vi "MC_7_12b_JW.vi"() -> ()   [LabVIEW 2011]
uses:
  <vilib>/Utility/file.llb/Read From Spreadsheet File (string).vi
  <vilib>/regexp/Match Regular Expression.xnode
  <vilib>/Utility/file.llb/Write To Spreadsheet File (string).vi
  <vilib>/Utility/file.llb/Write To Spreadsheet File (DBL).vi
  <vilib>/Utility/inputDevices.llb/keyboardAcquire.vi
panel:
  out "Current \nRecord":string[](array[string])
  out "Transformer \nHeaders":string[](array[string])
  out "Current Device ID":string
  out "Column":string
  out "Row":string
  out "Concentration Recorded":string
  out "Solvent Recorded":string
  out "Method Recorded":string
  in  "?":T1(tab)
  out "Material Recorded":string
  in  "Treatment Concentration (mM):":dbl=30.0
  in  "Surface Treatment:":string
  in  "# Drops*:":dbl=inf
  in  "Solution Temp (C):":dbl=55.0
  in  "Relative Humidity (%):":dbl=nan
  in  "Room Temp (F):":dbl=nan
  in  "Time (s):":dbl=80.0
  out "Accel (RPM/s):":dbl
  in  "RPM:":dbl=1000.0
  in  "Wait Time (s):":dbl=10.0
  in  "Sample #:":dbl=1.0
  in  "Fabricator:":string="Jeremy"
  in  "Data File":path
  out "Data Folder":path
  in  "Image Folder":path
  out "Image File":path=path "D:/UserData/Desktop/Jeremy/WFU/Research/Programs/VI mods/Image Not Found.png"
  in  "Ramp (s):":dbl=3.0
  out "Cal: Trap Density-STS":dbl format="%#_4e"
  out "New: Trap Density-STS":dbl format="%#_4e"
  out "Rec: Trap Density-STS":dbl caption="Trap Density-STS" format="%#_4e"
  out "Cal: Trap Density-VT":dbl format="%#_4e"
  out "New: Trap Density-VT":dbl format="%#_4e"
  out "Rec: Trap Density-VT":dbl caption="Trap Density-VT" format="%#_4e"
  out "Calc: Onset V":dbl
  out "New: Onset":dbl
  out "Rec: Onset V":dbl caption="Onset V"
  out "Cal: Mobility-Lin":dbl format="%#_4e"
  out "New: Mobility-Lin":dbl format="%#_4e"
  out "Rec: Mobility-Lin":dbl caption="Mobility-Lin" format="%#_4e"
  out "Cal: Mobility-Sat":dbl format="%#_4e"
  out "Rec: Length":dbl caption="Length"
  out "Width":dbl
  out "Rec: Dielectric (d)":dbl caption="Dielectric (d)"
  out "XY Graph":cluster{dbl[], dbl[]}[](graph)
  in  "NumPts":dbl=5.0
  in  "Cancel Button":bool
  in  "Next Button":bool
  in  "Previous Button":bool
  in  "Up Button":bool
  in  "Down Button":bool
  out "Data Name":string
  in  "Save Changes?":bool
  in  "New Dielectric":dbl
  in  "New Length":dbl
  in  "New Width":dbl
  out "New: Mobility-Sat":dbl format="%#_4e"
  in  "Slide":dbl(slide) step=1.0 scale=-14.3..84.0 scale format="%#_1p"
  in  "Blank Button":bool
  in  "Zoom":i16(slide)=-3 scale=-5.0..5.0
  out "Image Out 2":T2(plugin-control)
  out "Image Out":T2(plugin-control)
  in  "Magnification":u16(ring) items=["5x", "10x", "20x", "50x", "80x"]
  out "Total Width":dbl
  out "Distances":dbl[](array[numeric])
  in  "Undo Button":bool
  in  "Remove Button":bool
  out "Rec: Mobility-Sat":dbl caption="Mobility-Sat" format="%#_4e"
  out "Index":string
  out "Image Name":string
  in  "Export":bool
  out "Calc: VT":dbl
  out "New: VT":dbl
  in  "Manual":bool
  out "XY Graph 2":cluster{dbl[], dbl[]}[](graph)
  in  "Next Button 2":bool
  in  "Previous Button 2":bool
  in  "Slide 2":dbl(slide) step=1.0 scale=-1.0..82.0 scale format="%#_1p"
  out "Calc: STS":dbl
  out "New: STS":dbl
  in  "NumPts 2":dbl=5.0 caption="NumPts"
  out "Rec: VT":dbl caption="Threshold V"
  out "Rec: STS":dbl caption="STS"
  out "Rec: On/Off":dbl caption="On/Off" format="%#_3e"
  in  "Save Changes? 2":bool
  in  "Save Changes? 3":bool
  out "Date Recorded":string="Date Recorded"
  out "String":string
  in  "No Image":path=path "D:/UserData/Desktop/Jeremy/WFU/Research/Programs/VI mods/Image Not Found.png"
  in  "Project":path=path "D:/UserData/Desktop/Jeremy/WFU/Research/Programs/Mega Awesome/DeviceData.opj"
  out "Index 2":dbl
  out "Array 8":dbl[](array[numeric])
  out "Array 7":dbl[](array[numeric])
  out "ROI Descriptor out":T3 {"Contours"."Type" items=["No Selection", "Point", "Line", "Rectangle", "Oval", "Polygon", "Freehand Region", "Annulus", "Unused2", "Unused3", "Broken Line", "Freehand Line", "Rotated Rectangle"]}
  out "ROI Descriptor":T3 {"Contours"."Type" items=["No Selection", "Point", "Line", "Rectangle", "Oval", "Polygon", "Freehand Region", "Annulus", "Unused2", "Unused3", "Broken Line", "Freehand Line", "Rotated Rectangle"]}
  out "Numeric 3":dbl
  out "Array 6":dbl[][](array[numeric])
  out "Cluster":T4
  out "Array 5":dbl[](array[numeric])
  out "Array 4":dbl[](array[numeric])
  out "Array 3":dbl[](array[numeric])
  out "Numeric 2":dbl
  out "Numeric":dbl
  out "Array 2":dbl[](array[numeric])
  out "Array":dbl[](array[numeric])
  out "Index":dbl
  out "Table Control 2":string[][](table)
  out "Table Control":string[][](table)
  in  "Row Start":dbl=20.0
  # "Data Locations"
  # "Data Location"
  # "Image Location"
  # "Sample Properties"
  # "*     Inf = Full coverage\n   NaN = Unknown or Not Applicable"
  # "Recorded"
  # "Calculated"
  # "Re-Calculated"
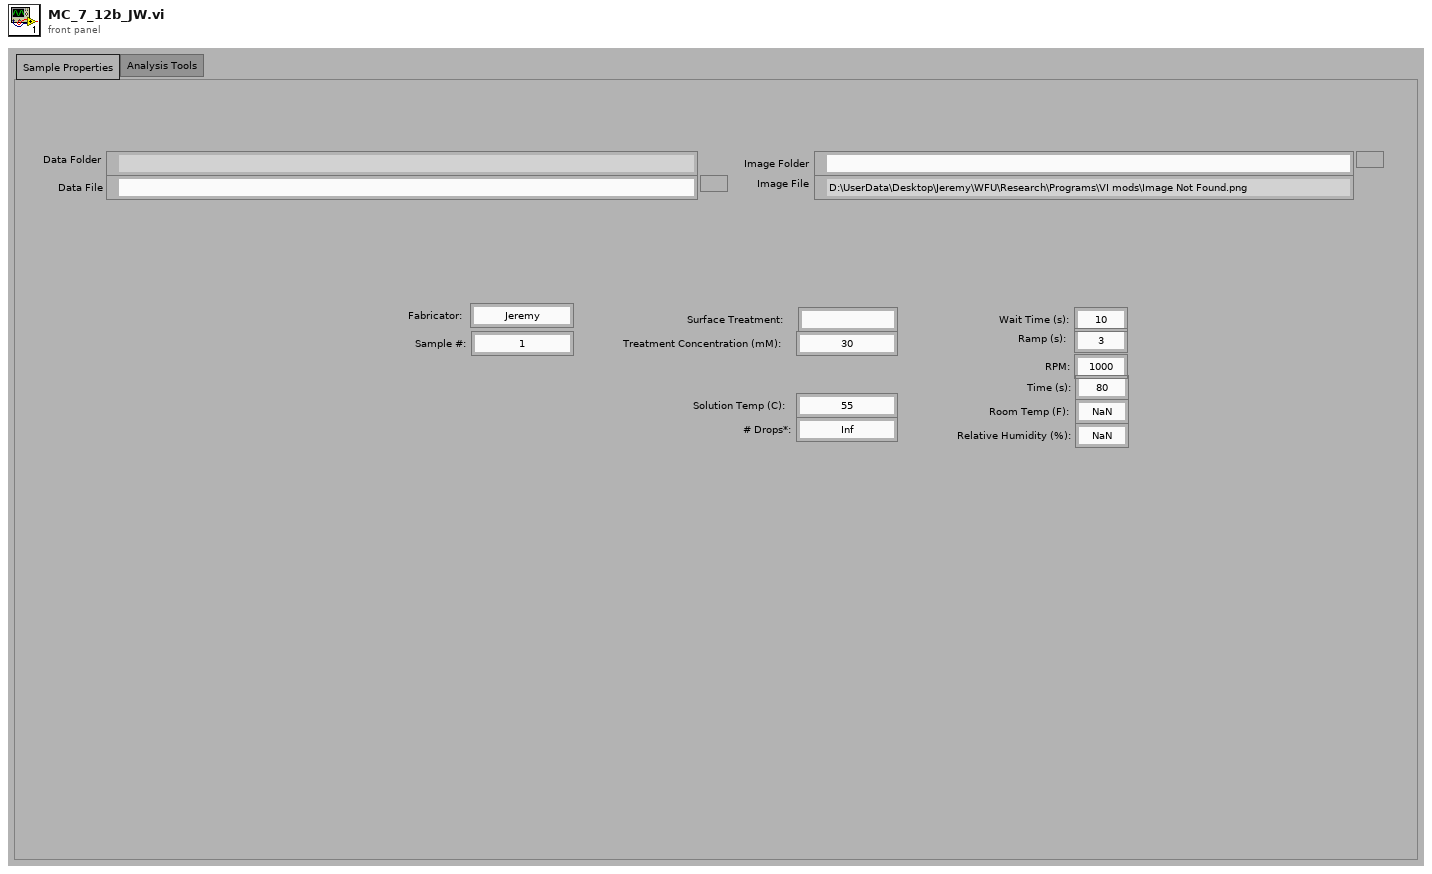
[diagram p1: front panel]
types:
  T1 = enum32{"Sample Properties", "Analysis Tools", "Current Database"}
  T2 = typedef "IMAQ Image.ctl" = refnum<image>
  T3 = typedef "ROI Descriptor" = cluster{"Global Rectangle":i32[], "Contours":cluster{"ID":enum32{"External", "Internal"}, "Type":u32, "Coordinates":i32[]}[]}
  T4 = cluster{"Numeric":dbl, "Numeric 2":dbl, "Numeric 3":dbl, "Numeric 4":dbl}
  T5 = cluster{"[0]":cluster{dbl[], dbl[]}, "[1]":cluster{dbl[], dbl[]}, "[2]":cluster{dbl[], dbl[]}, "[3]":cluster{dbl[], dbl[]}, "[4]":cluster{dbl[], dbl[]}, "[5]":cluster{dbl[], dbl[]}, "[6]":cluster{dbl[], dbl[]}, "[7]":cluster{dbl[], dbl[]}, "[8]":cluster{dbl[], dbl[]}}
  T6 = cluster{"Global Rectangle":i32[], "Contours":cluster{"Contour Type":u32, "ROI Type":u32, "Points":i32[]}[]}
  T7 = typedef "LVBoundsTypeDef.ctl" = cluster{"Width":u32, "Height":u32}
  T8 = enum16{"0", "1", "2", "3", "4", "5", "6", "7", "8", "9", "A", "B", "C", "D", "E", "F", "G", "H", "I", "J", "K", "L", "M", "N", "O", "P", "Q", "R", "S", "T", "U", "V", "W", "X", "Y", "Z", "F1", "F2", "F3", "F4", "F5", "F6", "F7", "F8", "F9", "F10", "F11", "F12", "F13", "F14", "F15", "ADD", "BACK", "BACKSLASH", "CAPITAL", "COMMA", "DECIMAL", "DELETE", "DIVIDE", "DOWN", "END", "EQUALS", "ESCAPE", "GRAVE (`)", "HOME", "INSERT", "LBRACKET", "LCONTROL", "LEFT", "L ALT", "LSHIFT", "LWIN", "MINUS", "MULTIPLY", "NEXT", "NUMLOCK", "NUMPAD_0", "NUMPAD_1", "NUMPAD_2", "NUMPAD_3", "NUMPAD_4", "NUMPAD_5", "NUMPAD_6", "NUMPAD_7", "NUMPAD_8", "NUMPAD_9", "PAUSE", "PERIOD", "PRIOR (PG UP)", "RBRACKET", "RCONTROL", "RETURN", "RIGHT", "R ALT", "RSHIFT", "RWIN", "SCROLL", "SEMICOLON", "SLASH", "SPACE", "SUBTRACT", "TAB", "UP", "ENTER (num pad)", "' (quote)"}[]
  T9 = cluster{"Contour Type":u32, "ROI Type":u32, "Points":i32[]}[]
  T10 = cluster{i32[], cluster{"Contour Type":u32, "ROI Type":u32, "Points":i32[]}[]}
  T11 = enum16{"0", "1", "2", "3", "4", "5", "6", "7", "8", "9", "A", "B", "C", "D", "E", "F", "G", "H", "I", "J", "K", "L", "M", "N", "O", "P", "Q", "R", "S", "T", "U", "V", "W", "X", "Y", "Z", "F1", "F2", "F3", "F4", "F5", "F6", "F7", "F8", "F9", "F10", "F11", "F12", "F13", "F14", "F15", "ADD", "BACK", "BACKSLASH", "CAPITAL", "COMMA", "DECIMAL", "DELETE", "DIVIDE", "DOWN", "END", "EQUALS", "ESCAPE", "GRAVE (`)", "HOME", "INSERT", "LBRACKET", "LCONTROL", "LEFT", "L ALT", "LSHIFT", "LWIN", "MINUS", "MULTIPLY", "NEXT", "NUMLOCK", "NUMPAD_0", "NUMPAD_1", "NUMPAD_2", "NUMPAD_3", "NUMPAD_4", "NUMPAD_5", "NUMPAD_6", "NUMPAD_7", "NUMPAD_8", "NUMPAD_9", "PAUSE", "PERIOD", "PRIOR (PG UP)", "RBRACKET", "RCONTROL", "RETURN", "RIGHT", "R ALT", "RSHIFT", "RWIN", "SCROLL", "SEMICOLON", "SLASH", "SPACE", "SUBTRACT", "TAB", "UP", "ENTER (num pad)", "' (quote)"}
  T12 = cluster{string, sgl, bool, bool, bool, bool, bool, bool, i32}
  T13 = cluster{i32, cluster{string, sgl, bool, bool, bool, bool, bool, bool, i32}, i32, i32}
  T14 = cluster{"Contour Type":u32, "ROI Type":u32, "Points":i32[]}
  T15 = cluster{"Points[0]":i32, "Points[1]":i32, "Points[2]":i32, "Points[3]":i32, "Points[4]":i32, "Points[5]":i32, "Points[6]":i32, "Points[7]":i32, "Points[8]":i32}
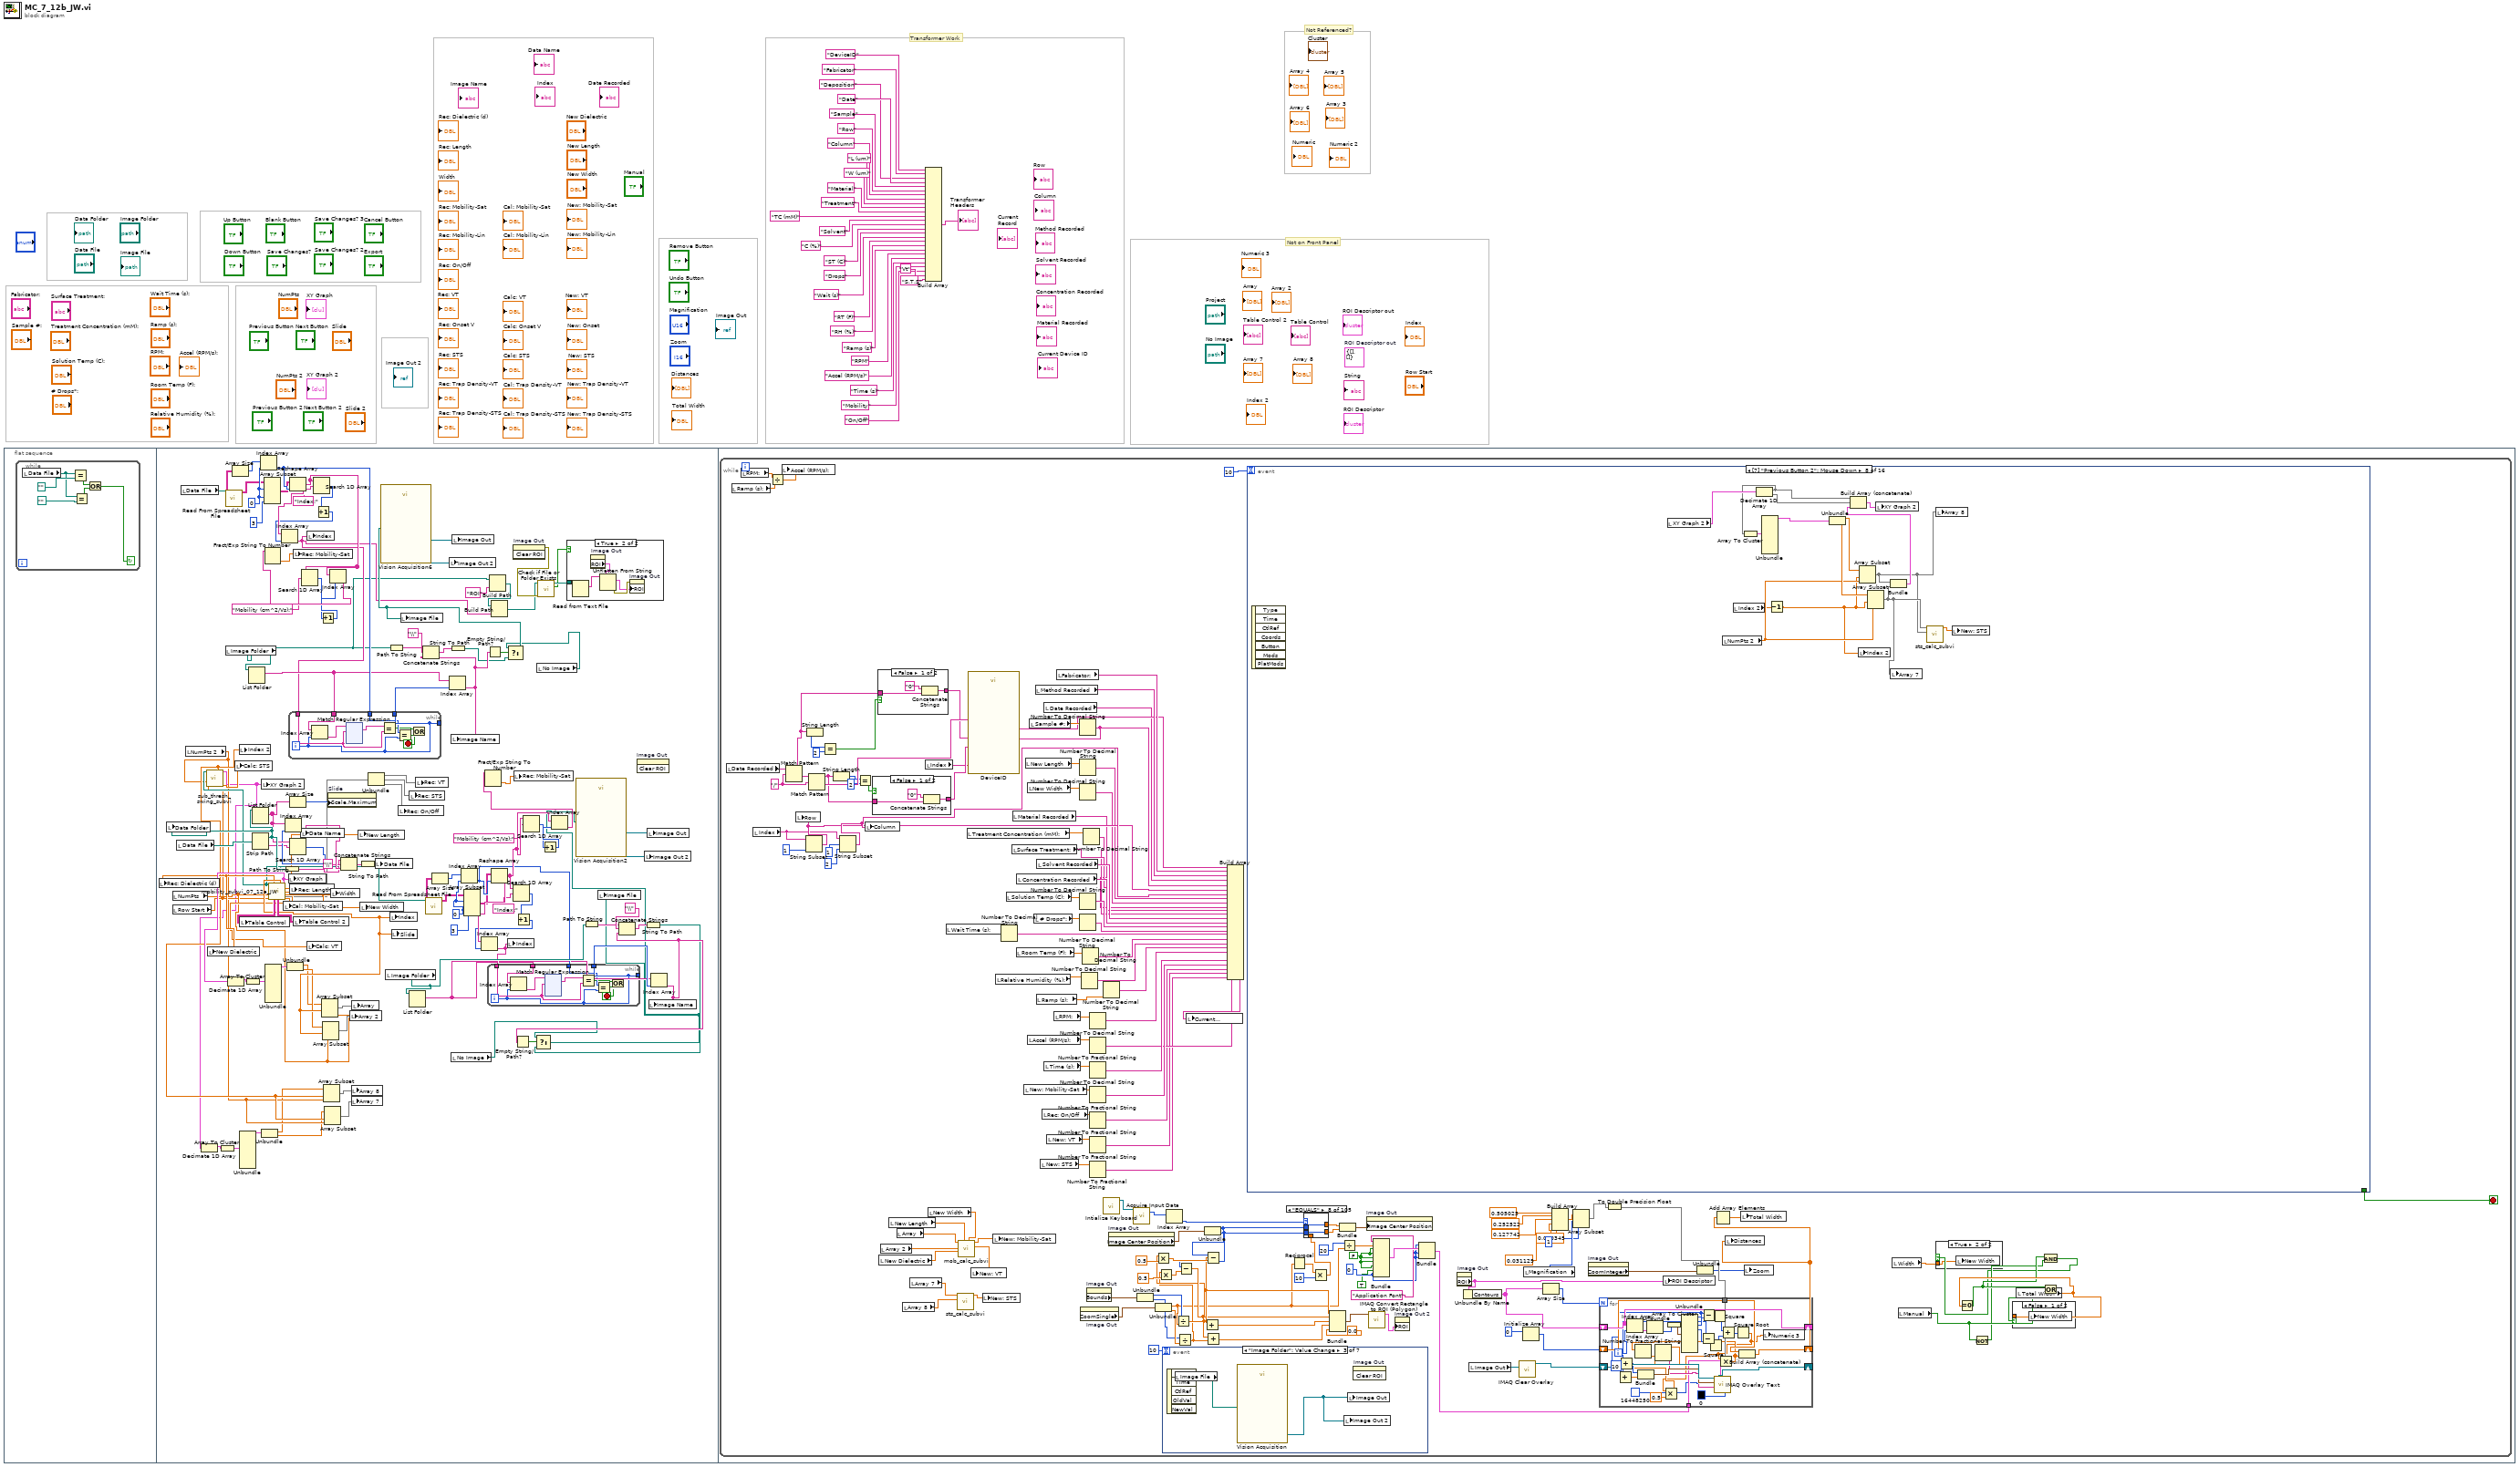
[diagram p0: block diagram]
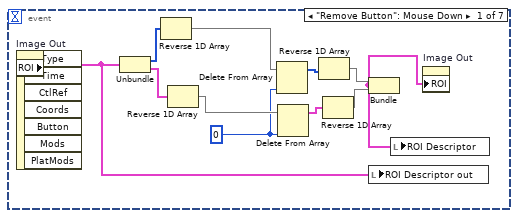
[diagram p7: hidden frame]
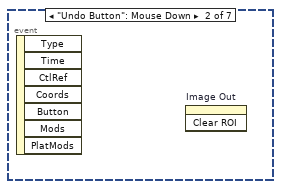
[diagram p8: hidden frame]
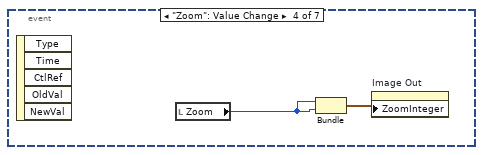
[diagram p9: hidden frame]
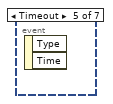
[diagram p10: hidden frame]
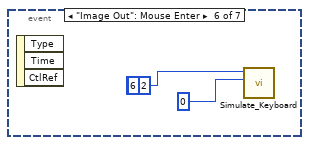
[diagram p11: hidden frame]
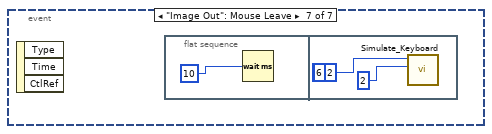
[diagram p12: hidden frame]
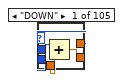
[diagram p13: hidden frame]
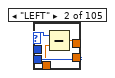
[diagram p14: hidden frame]
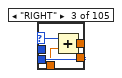
[diagram p15: hidden frame]
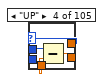
[diagram p16: hidden frame]
diagram:
  (unwired) T3 {"Global Rectangle"=[], "Contours"=[]}  # ROI Descriptor out
  # "Not Referenced?"
  # "Transformer Work"
  # "Not on Front Panel"
  n1 = flat-sequence {
    frame #0 {
      n2 = while {
        stop <- w29 continue-if-true
        n3 = local read "Data File"() -> (w31:path)
        n4 = Equal?(x=w31, y=path "") -> (x = y?=w33:bool)
        n5 = Equal?(x=w31, y=path "") -> (x = y?=w32:bool)
        n6 = Or(x=w33, y=w32) -> (x .or. y?=w29:bool)
      }
    }
    frame #1 {
      w95 = 0
      w125 = 0
      n7 = local read "NumPts"() -> (w70:dbl)
      n8 = local read "Row Start"() -> (w69:dbl)
      n9 = local read "Data File"() -> (w99:path)
      n10 = local read "Data File"() -> (w120:path)
      n11 = local read "NumPts 2"() -> (w64:dbl)
      n12 = call-poly <vilib>:"Read From Spreadsheet File.vi"("file path (dialog if empty)"=w120) -> ("all rows"=w123:string[][])  [unwired: 6 in, 4 out]
      n13 = local read "Image Folder"() -> (w35:path)
      n14 = Array Size(array=w123) -> (size(s)=w124:i32[])
      n15 = List Folder(path=w35) -> (filenames=w129:string[])  [unwired: 3 in, 3 out]
      n16 = Strip Path(path=w99) -> (stripped path=w100:path, name=w81:string)
      n17 = local write "Data Folder"(w100) -> ()
      n18 = List Folder(path=w100) -> (filenames=w89:string[])  [unwired: 3 in, 3 out]
      n19 = Index Array(array=w124, index=w125) -> (element=w131:i32)
      n20 = Array Subset(array=w123, index (row)=w125, index (col)=w125, length (col)=3) -> (w122:string[][])  [unwired: 1 in]
      n21 = Path To String(path=w100) -> (string=w80:string)
      n22 = Reshape Array(w122, w131) -> (w141:string[])
      n23 = Array Size(array=w89) -> (size(s)=w90:i32)
      n24 = Search 1D Array(1D array=w89, element=w81) -> (index of element=w88:i32)  [unwired: 1 in]
      n25 = Index Array(array=w89, index=w88) -> (element=w87:string)
      n26 = local write "Data Name"(w87) -> ()
      n27 = Search 1D Array(1D array=w141, element="Mobility (cm^2/Vs):") -> (index of element=w136:i32)  [unwired: 1 in]
      n28 = Search 1D Array(1D array=w141, element="Index:") -> (index of element=w128:i32)  [unwired: 1 in]
      n29 = Increment(x=w128) -> (x+1=w127:i32)
      n30 = Index Array(array=w141, index=w127) -> (element=w36:string)
      n31 = while {
        tunnel: w129 -> [w274]
        tunnel: w36 -> [w272]
        tunnel: [w271] -> _
        tunnel: [w271] -> w130
        tunnel: w131 -> [w270]
        i -> [w271]
        stop <- w267 stop-if-true
        n32 = Index Array(array=w274, index=w271) -> (element=w275:string)
        n33 = xnode "Match Regular Expression"("input string"=w275, "regular expression"=w272) -> ("whole match"=w273:string)  [unwired: 4 in, 4 out]
        n34 = Equal?(x=w273, y=w272) -> (x = y?=w269:bool)
        n35 = Equal?(x=w270, y=w271) -> (x = y?=w268:bool)
        n36 = Or(x=w269, y=w268) -> (x .or. y?=w267:bool)
      }
      n37 = local write "Index"(w36) -> ()
      n38 = Increment(x=w136) -> (x+1=w137:i32)
      n39 = property on="Slide" class="Slide (strict)"("Scale.Maximum"=w90) -> ()  [unwired: 2 in, 2 out]
      n40 = Index Array(array=w141, index=w137) -> (element=w139:string)
      n41 = Fract/Exp String To Number(string=w139) -> (number=w140:dbl)  [unwired: 3 in, 1 out]
      n42 = local write "Rec: Mobility-Sat"(w140) -> ()
      n43 = Concatenate Strings(w80, "\\", w87) -> (w82:string)
      n44 = String To Path(string=w82) -> (path=w71:path)
      n45 = call "sub_thresh_swing_subvi.vi"("Path"=w71, "NumPts"=w64, "Row Start"=w69) -> ("Index"=w65:dbl, "XY Graph"=w60:cluster{dbl[], dbl[]}[], "Sub Threshold Swing"=w72:dbl)  [unwired: 8 in, 2 out]
      n46 = Decimate 1D Array(w60) -> (w61:cluster{dbl[], dbl[]}[])  [unwired: 1 out]
      n47 = Array To Cluster(array=w61) -> (cluster=w63:T5)
      n48 = local write "Calc: STS"(w72) -> ()
      n49 = local write "Index 2"(w65) -> ()
      n50 = Unbundle(w63) -> ("[0]"=w62:cluster{dbl[], dbl[]})  [unwired: 8 out]
      n51 = local write "XY Graph 2"(w60) -> ()
      n52 = Unbundle(w62) -> (w58:dbl[], w57:dbl[])
      n53 = call "mobility_subvi_07_12a_JW.vi"("Path"=w71, "NumPts"=w70, 11:w69) -> ("Dielectric (d)"=w76:dbl, "Index"=w77:dbl, "XY Graph"=w119:cluster{dbl[], dbl[]}[], "Length"=w75:dbl, "Vt"=w73:dbl, "Width"=w74:dbl, "Table Control"=w84:string[][], "Table Control 2"=w85:string[][], 14:w54, "Mobility"=w86:dbl)  [unwired: 2 in, 1 out]
      n54 = local write "Rec: Dielectric (d)"(w76) -> ()
      n55 = local write "New Dielectric"(w76) -> ()
      n56 = Decimate 1D Array(w119) -> (w118:cluster{dbl[], dbl[]}[])  [unwired: 1 out]
      n57 = local write "Table Control"(w84) -> ()
      n58 = Array To Cluster(array=w118) -> (cluster=w116:T5)
      n59 = Unbundle(w116) -> ("[0]"=w117:cluster{dbl[], dbl[]})  [unwired: 8 out]
      n60 = local write "Cal: Mobility-Sat"(w86) -> ()
      n61 = Unbundle(w117) -> (w59:dbl[], w66:dbl[])
      n62 = local write "XY Graph"(w119) -> ()
      n63 = local write "Rec: Length"(w75) -> ()
      n64 = local write "Table Control 2"(w85) -> ()
      n65 = local write "Calc: VT"(w73) -> ()
      n66 = Array Subset(array=w59, index=w77, length=w70) -> (w78:dbl[])
      n67 = Array Subset(array=w66, index=w77, length=w70) -> (w79:dbl[])
      n68 = Array Subset(array=w58, index=w65, length=w64) -> (w68:dbl[])
      n69 = Array Subset(array=w57, index=w65, length=w64) -> (w67:dbl[])
      n70 = local write "Width"(w74) -> ()
      n71 = local write "Array 2"(w79) -> ()
      n72 = local write "Array 8"(w68) -> ()
      n73 = local write "Array 7"(w67) -> ()
      n74 = local write "Array"(w78) -> ()
      n75 = local write "New Length"(w75) -> ()
      n76 = local write "New Width"(w74) -> ()
      n77 = Unbundle(w54) -> ("Vt"=w56, "STS"=w55, "On/Off"=w53)
      n78 = local write "Data File"(w71) -> ()
      n79 = local read "Image Folder"() -> (w106:path)
      n80 = Path To String(path=w35) -> (string=w133:string)
      n81 = local write "Index"(w77) -> ()
      n82 = local write "Slide"(w77) -> ()
      n83 = local write "Rec: On/Off"(w53) -> ()
      n84 = List Folder(path=w106) -> (filenames=w102:string[])  [unwired: 3 in, 3 out]
      n85 = local write "Rec: STS"(w55) -> ()
      n86 = local write "Rec: VT"(w56) -> ()
      n87 = call-poly <vilib>:"Read From Spreadsheet File.vi"("file path (dialog if empty)"=w71) -> ("all rows"=w93:string[][])  [unwired: 6 in, 4 out]
      n88 = Array Size(array=w93) -> (size(s)=w94:i32[])
      n89 = Index Array(array=w129, index=w130) -> (element=w52:string)
      n90 = Concatenate Strings(w133, "\\", w52) -> (w134:string)
      n91 = String To Path(string=w134) -> (path=w50:path)
      n92 = local write "Image Name"(w52) -> ()
      n93 = local read "No Image"() -> (w44:path)
      n94 = Index Array(array=w94, index=w95) -> (element=w105:i32)
      n95 = Array Subset(array=w93, index (row)=w95, index (col)=w95, length (col)=3) -> (w92:string[][])  [unwired: 1 in]
      n96 = Empty String/Path?(string/path=w52) -> (empty?=w51:bool)
      n97 = Build Path(base path=w35, name or relative path="ROI") -> (appended path=w38:path)
      n98 = Build Path(base path=w38, name or relative path=w36) -> (appended path=w37:path)
      n99 = Reshape Array(w92, w105) -> (w115:string[])
      n100 = invoke on="Image Out" class="ImageControl" method="Clear ROI"() -> (error out=w42:errorcluster)  [unwired: 3 in, 2 out]
      n101 = Search 1D Array(1D array=w115, element="Index:") -> (index of element=w98:i32)  [unwired: 1 in]
      n102 = Increment(x=w98) -> (x+1=w97:i32)
      n103 = Index Array(array=w115, index=w97) -> (element=w103:string)
      n104 = while {
        tunnel: w102 -> [w154]
        tunnel: w103 -> [w152]
        tunnel: [w151] -> _
        tunnel: [w151] -> w104
        tunnel: w105 -> [w150]
        i -> [w151]
        stop <- w147 stop-if-true
        n105 = Index Array(array=w154, index=w151) -> (element=w155:string)
        n106 = xnode "Match Regular Expression"("input string"=w155, "regular expression"=w152) -> ("whole match"=w153:string)  [unwired: 4 in, 4 out]
        n107 = Equal?(x=w153, y=w152) -> (x = y?=w149:bool)
        n108 = Equal?(x=w150, y=w151) -> (x = y?=w148:bool)
        n109 = Or(x=w149, y=w148) -> (x .or. y?=w147:bool)
      }
      n110 = local write "Index"(w103) -> ()
      n111 = Search 1D Array(1D array=w115, element="Mobility (cm^2/Vs):") -> (index of element=w110:i32)  [unwired: 1 in]
      n112 = local read "No Image"() -> (w43:path)
      n113 = Select(t=w43, s=w51, f=w50) -> (s? t:f=w49:path)
      n114 = call "Vision Acquisition6"("Image Path"=w49) -> ("Image Out"=w132:T2)  [unwired: 25 in, 1 out]
      n115 = local write "Image File"(w49) -> ()
      n116 = local write "Image Out 2"(w132) -> ()
      n117 = local write "Image Out"(w132) -> ()
      n118 = call <vilib>:"Check if File or Folder Exists.vi"("error in (no error)"=w42, "path"=w37) -> ("file or folder exists?"=w40:bool, "dup path"=w41:path)  [unwired: 7 in, 1 out]
      n119 = Increment(x=w110) -> (x+1=w111:i32)
      n120 = Index Array(array=w115, index=w111) -> (element=w113:string)
      n121 = Fract/Exp String To Number(string=w113) -> (number=w114:dbl)  [unwired: 3 in, 1 out]
      n122 = local write "Rec: Mobility-Sat"(w114) -> ()
      n123 = case shown="True" w40 {
        tunnel: w41 -> [_ w142]
        frame False {
        }
        frame True {
          n124 = Read from Text File(file (use dialog)=w142) -> (text=w146:string)  [unwired: 3 in, 3 out]
          n125 = property on="Image Out" class="ImageControl"() -> ("ROI"=w143:T6)  [unwired: 2 in, 2 out]
          n126 = Unflatten From String(type=w143, binary string=w146) -> (value=w144:T6, error out=w145:errorcluster)  [unwired: 3 in, 1 out]
          n127 = property on="Image Out" class="ImageControl"(error in=w145, "ROI"=w144) -> ()  [unwired: 1 in, 2 out]
        }
      }
      n128 = Path To String(path=w106) -> (string=w107:string)
      n129 = invoke on="Image Out" class="ImageControl" method="Clear ROI"() -> ()  [unwired: 3 in, 3 out]
      n130 = Index Array(array=w102, index=w104) -> (element=w47:string)
      n131 = Empty String/Path?(string/path=w47) -> (empty?=w48:bool)
      n132 = Concatenate Strings(w107, "\\", w47) -> (w108:string)
      n133 = String To Path(string=w108) -> (path=w46:path)
      n134 = Select(t=w44, s=w48, f=w46) -> (s? t:f=w45:path)
      n135 = call "Vision Acquisition2"("Image Path"=w45) -> ("Image Out"=w101:T2)  [unwired: 25 in, 1 out]
      n136 = local write "Image File"(w45) -> ()
      n137 = local write "Image Out 2"(w101) -> ()
      n138 = local write "Image Out"(w101) -> ()
      n139 = local write "Image Name"(w47) -> ()
    }
    frame #2 {
      n140 = while {
        stop <- w533 stop-if-true
        w419 = "/"
        w483 = FALSE
        w481 = 0
        n141 = local read "Date Recorded"() -> (w422:string)
        n142 = local read "Ramp (s):"() -> (w388:dbl)
        n143 = local read "RPM:"() -> (w389:dbl)
        n144 = local read "Index"() -> (w391:string)
        n145 = Divide(x=w389, y=w388) -> (x/y=w387:dbl)
        n146 = local write "Accel (RPM/s):"(w387) -> ()
        n147 = Match Pattern(string=w422, regular expression=w419) -> (before substring=w413:string, after substring=w420:string)  [unwired: 1 in, 2 out]
        n148 = String Subset(string=w391, length (rest)=1) -> (substring=w447:string)  [unwired: 1 in]
        n149 = local write "Row"(w447) -> ()
        n150 = String Length(string=w413) -> (length=w416:i32)
        n151 = Match Pattern(string=w420, regular expression=w419) -> (before substring=w407:string, after substring=w418:string)  [unwired: 1 in, 2 out]
        n152 = Equal?(x=w416, y=2) -> (x = y?=w414:bool)
        n153 = String Length(string=w407) -> (length=w409:i32)
        n154 = String Subset(string=w391, offset (0)=1, length (rest)=2) -> (substring=w448:string)
        n155 = Equal?(x=w409, y=2) -> (x = y?=w411:bool)
        n156 = local write "Column"(w448) -> ()
        n157 = case shown="False" w411 {
          tunnel: w407 -> [w535 w537]
          tunnel: [w534 w537] -> w408
          frame False {
            n158 = Concatenate Strings("0", w535) -> (w534:string)
          }
          frame True {
          }
        }
        n159 = case shown="False" w414 {
          tunnel: w413 -> [w539 w541]
          tunnel: [w538 w541] -> w412
          frame False {
            n160 = Concatenate Strings("0", w539) -> (w538:string)
          }
          frame True {
          }
        }
        n161 = local read "New Dielectric"() -> (w471:dbl)
        n162 = local read "Array 2"() -> (w467:dbl[])
        n163 = local read "New Length"() -> (w469:dbl)
        n164 = local read "Array"() -> (w468:dbl[])
        n165 = local read "Array 8"() -> (w463:dbl[])
        n166 = local read "Array 7"() -> (w464:dbl[])
        n167 = local read "Index"() -> (w406:string)
        n168 = local read "New Width"() -> (w472:dbl)
        n169 = local read "Wait Time (s):"() -> (w452:dbl)
        n170 = call "sts_calc_subvi.vi"("Array 2"=w463, "Array"=w464) -> ("STS"=w465:dbl)  [unwired: 9 in]
        n171 = call "mob_calc_subvi.vi"("Width"=w472, "Length"=w469, "Dielectric (d)"=w471, "Array 2"=w467, "Array"=w468) -> ("Vt"=w466:dbl, "Mobility"=w470:dbl)  [unwired: 4 in, 1 out]
        n172 = local read "Treatment Concentration (mM):"() -> (w399:dbl)
        n173 = local write "New: VT"(w466) -> ()
        n174 = local write "New: STS"(w465) -> ()
        n175 = local write "New: Mobility-Sat"(w470) -> ()
        n176 = local read "Relative Humidity (%):"() -> (w396:dbl)
        n177 = Number To Decimal String(number=w452) -> (decimal integer string=w453:string)  [unwired: 1 in]
        n178 = local read "Solution Temp (C):"() -> (w441:dbl)
        n179 = local read "Surface Treatment:"() -> (w398:string)
        n180 = local read "Material Recorded"() -> (w394:string)
        n181 = local read "Room Temp (F):"() -> (w445:dbl)
        n182 = local read "Concentration Recorded"() -> (w401:string)
        n183 = local read "New: Mobility-Sat"() -> (w434:dbl)
        n184 = local read "New Length"() -> (w405:dbl)
        n185 = local read "New Width"() -> (w404:dbl)
        n186 = local read "Accel (RPM/s):"() -> (w432:dbl)
        n187 = local read "Sample #:"() -> (w424:dbl)
        n188 = local read "# Drops*:"() -> (w442:dbl)
        n189 = local read "Method Recorded"() -> (w425:string)
        n190 = local read "Ramp (s):"() -> (w450:dbl)
        n191 = local read "Solvent Recorded"() -> (w400:string)
        n192 = local read "New: STS"() -> (w426:dbl)
        n193 = local read "Rec: On/Off"() -> (w430:dbl)
        n194 = local read "Date Recorded"() -> (w421:string)
        n195 = local read "Time (s):"() -> (w437:dbl)
        n196 = local read "New: VT"() -> (w428:dbl)
        n197 = local read "RPM:"() -> (w438:dbl)
        n198 = local read "Fabricator:"() -> (w446:string)
        n199 = Number To Decimal String(number=w442) -> (decimal integer string=w443:string)  [unwired: 1 in]
        n200 = Number To Decimal String(number=w424) -> (decimal integer string=w417:string)  [unwired: 1 in]
        n201 = call "DeviceID"("Sample"=w417, "Year"=w418, "Month"=w412, "Day"=w408, "Index"=w406) -> ("Result"=w423:string)  [unwired: 9 in, 1 out]
        n202 = Number To Decimal String(number=w405) -> (decimal integer string=w403:string)  [unwired: 1 in]
        n203 = Number To Decimal String(number=w404) -> (decimal integer string=w402:string)  [unwired: 1 in]
        n204 = Number To Decimal String(number=w441) -> (decimal integer string=w440:string)  [unwired: 1 in]
        n205 = property on="Image Out" class="ImageControl"() -> ("ZoomSingle"=w501:cluster{"X":sgl, "Y":sgl})  [unwired: 2 in, 2 out]
        n206 = Number To Decimal String(number=w396) -> (decimal integer string=w395:string)  [unwired: 1 in]
        n207 = Number To Decimal String(number=w445) -> (decimal integer string=w444:string)  [unwired: 1 in]
        n208 = Number To Decimal String(number=w399) -> (decimal integer string=w397:string)  [unwired: 1 in]
        n209 = property on="Image Out" class="ImageControl"() -> ("Bounds"=w502:T7)  [unwired: 2 in, 2 out]
        n210 = Number To Decimal String(number=w438) -> (decimal integer string=w439:string)  [unwired: 1 in]
        n211 = Number To Fractional String(number=w432) -> (F-format string=w433:string)  [unwired: 3 in]
        n212 = Number To Decimal String(number=w437) -> (decimal integer string=w436:string)  [unwired: 1 in]
        n213 = Number To Fractional String(number=w434) -> (F-format string=w435:string)  [unwired: 3 in]
        n214 = Number To Fractional String(number=w430) -> (F-format string=w431:string)  [unwired: 3 in]
        n215 = Number To Fractional String(number=w428) -> (F-format string=w429:string)  [unwired: 3 in]
        n216 = Number To Fractional String(number=w426) -> (F-format string=w427:string)  [unwired: 3 in]
        n217 = Number To Decimal String(number=w450) -> (decimal integer string=w451:string)  [unwired: 1 in]
        n218 = call <vilib>:"Intialize Keyboard.vi"() -> ("device ID"=w513:refnum<k1>)  [unwired: 10 in, 1 out]
        n219 = property on="Image Out" class="ImageControl"() -> ("Image Center Position"=w508:cluster{"X":u32, "Y":u32})  [unwired: 2 in, 2 out]
        n220 = call-poly <vilib>:"Acquire Input Data.vi"("device ID"=w513) -> ("keys pressed"=w512:T8)  [unwired: 16 in, 2 out]
        n221 = Unbundle(w502) -> ("Width"=w499:u32, "Height"=w498:u32)
        n222 = Unbundle(w501) -> ("X"=w476:sgl, "Y"=w500:sgl)
        n223 = event shown="[2] \" Image Folder\": Value Change" {
          selector: _ -> [_ _ _ _ _ _ _]
          dyn-events: _ -> [_ _ _ _ _ _ _]
          timeout: 10 -> [_ _ _ _ _ _ _]
          event "Remove Button": Mouse Down {
            w546 = 0
            n224 = property on="Image Out" class="ImageControl"() -> ("ROI"=w544:T6)  [unwired: 2 in, 2 out]
            n225 = event-data() -> ()  [unwired: 1 in, 7 out]
            n226 = Unbundle(w544) -> ("Global Rectangle"=w547:i32[], "Contours"=w549:T9)
            n227 = Reverse 1D Array(array=w547) -> (reversed array=w548:i32[])
            n228 = Reverse 1D Array(array=w549) -> (reversed array=w550:T9)
            n229 = Delete From Array(array=w548, index=w546) -> (array with subset deleted=w551:i32[])  [unwired: 1 in, 1 out]
            n230 = Delete From Array(array=w550, index=w546) -> (array with subset deleted=w552:T9)  [unwired: 1 in, 1 out]
            n231 = Reverse 1D Array(array=w551) -> (reversed array=w553:i32[])
            n232 = Reverse 1D Array(array=w552) -> (reversed array=w554:T9)
            n233 = Bundle(w553, w554) -> (w545:T10)  [unwired: 1 in]
            n234 = local write "ROI Descriptor out"(w544) -> ()
            n235 = local write "ROI Descriptor"(w545) -> ()
            n236 = property on="Image Out" class="ImageControl"("ROI"=w545) -> ()  [unwired: 2 in, 2 out]
          }
          event "Undo Button": Mouse Down {
            n237 = event-data() -> ()  [unwired: 1 in, 7 out]
            n238 = invoke on="Image Out" class="ImageControl" method="Clear ROI"() -> ()  [unwired: 3 in, 3 out]
          }
          event "Image Folder": Value Change {
            n239 = event-data() -> ()  [unwired: 1 in, 5 out]
            n240 = local read "Image File"() -> (w556:path)
            n241 = call "Vision Acquisition"("Image Path"=w556) -> ("Image Out"=w555:T2)  [unwired: 25 in, 1 out]
            n242 = local write "Image Out 2"(w555) -> ()
            n243 = local write "Image Out"(w555) -> ()
            n244 = invoke on="Image Out" class="ImageControl" method="Clear ROI"() -> ()  [unwired: 3 in, 3 out]
          }
          event "Zoom": Value Change {
            n245 = event-data() -> ()  [unwired: 1 in, 5 out]
            n246 = local read "Zoom"() -> (w557:i16)
            n247 = Bundle("Zoom"=w557, "Zoom"=w557) -> (w558:cluster{"Zoom":i16, "Zoom":i16})  [unwired: 1 in]
            n248 = property on="Image Out" class="ImageControl"("ZoomInteger"=w558) -> ()  [unwired: 2 in, 2 out]
          }
          event Timeout {
            n249 = event-data() -> ()  [unwired: 1 in, 2 out]
          }
          event "Image Out": Mouse Enter {
            (unwired) 6
            n250 = event-data() -> ()  [unwired: 1 in, 3 out]
            n251 = call "Simulate_Keyboard.vi"("Action"=0, "Virtual Key"=162) -> ()  [unwired: 7 in, 1 out]
          }
          event "Image Out": Mouse Leave {
            n252 = event-data() -> ()  [unwired: 1 in, 3 out]
            n253 = flat-sequence {
              frame #0 {
                n254 = Wait (ms)(milliseconds to wait=10) -> ()  [unwired: 1 out]
              }
              frame #1 {
                (unwired) 6
                n255 = call "Simulate_Keyboard.vi"("Action"=2, "Virtual Key"=162) -> ()  [unwired: 7 in, 1 out]
              }
            }
          }
        }
        n256 = Index Array(array=w512) -> (element=w516:T11)  [unwired: 1 in]
        n257 = Divide(x=w499, y=w476) -> (x/y=w489:sgl)
        n258 = Multiply(x=w489, y=0.5) -> (x*y=w495:dbl)
        n259 = Divide(x=w498, y=w500) -> (x/y=w488:sgl)
        n260 = Multiply(x=w488, y=0.5) -> (x*y=w494:dbl)
        n261 = Unbundle(w508) -> ("X"=w490:u32, "Y"=w491:u32)
        n262 = Subtract(x=w491, y=w494) -> (x-y=w492:dbl)
        n263 = Subtract(x=w490, y=w495) -> (x-y=w493:dbl)
        n264 = Add(x=w493, y=w489) -> (x+y=w507:dbl)
        n265 = Add(x=w492, y=w488) -> (x+y=w506:dbl)
        n266 = Build Array(w423, w446, w425, w421, w417, w447, w448, w403, w402, w394, w398, w397, w400, w401, w440, w443, w453, w444, w395, w451, w439, w433, w436, w435, w431, w429, w427) -> (w449:string[])
        n267 = local write "Current \nRecord"(w449) -> ()
        n268 = event shown="[7] \"Previous Button 2\": Mouse Down" {
          selector: _ -> [_ _ _ _ _ _ _ _ _ _ _ _ _ _ _ _]
          dyn-events: _ -> [_ _ _ _ _ _ _ _ _ _ _ _ _ _ _ _]
          timeout: 10 -> [_ _ _ _ _ _ _ _ _ _ _ _ _ _ _ _]
          tunnel: [_ _ _ _ _ _ _ _ _ _ _ _ _ TRUE _ TRUE] -> w533
          event Timeout {
            n269 = event-data() -> ()  [unwired: 1 in, 2 out]
          }
          event "Down Button": Mouse Down {
            w889 = 0
            n270 = event-data() -> ()  [unwired: 1 in, 7 out]
            n271 = local read "NumPts 2"() -> (w850:dbl)
            n272 = local read "NumPts"() -> (w857:dbl)
            n273 = local read "Row Start"() -> (w856:dbl)
            n274 = local read "Data File"() -> (w894:path)
            n275 = property on="Image Out" class="ImageControl"() -> (error out=w819:errorcluster, "Image Center Position"=w823:cluster{"X":u32, "Y":u32})  [unwired: 2 in, 1 out]
            n276 = Strip Path(path=w894) -> (stripped path=w885:path, name=w907:string)
            n277 = local write "Data Folder"(w885) -> ()
            n278 = List Folder(path=w885) -> (filenames=w900:string[], error out=w828:errorcluster)  [unwired: 3 in, 2 out]
            n279 = Array Size(array=w900) -> (size(s)=w895:i32)
            n280 = Path To String(path=w885) -> (string=w908:string)
            n281 = Search 1D Array(1D array=w900, element=w907) -> (index of element=w897:i32)  [unwired: 1 in]
            n282 = Unbundle(w823) -> ("X"=w821:u32)  [unwired: 1 out]
            n283 = Bundle("X"=w821, 0) -> (w822:cluster{"X":u32, i32})  [unwired: 1 in]
            n284 = Decrement(x=w895) -> (x-1=w898:i32)
            n285 = Equal?(x=w897, y=w898) -> (x = y?=w899:bool)
            n286 = case shown="False" w899 {
              tunnel: w897 -> [w1035 _]
              tunnel: [w1034 0] -> w896
              frame False {
                n287 = Increment(x=w1035) -> (x+1=w1034:i32)
              }
              frame True {
              }
            }
            n288 = Index Array(array=w900, index=w896) -> (element=w901:string)
            n289 = local write "Data Name"(w901) -> ()
            n290 = Concatenate Strings(w908, "\\", w901) -> (w906:string)
            n291 = property on="Image Out" class="ImageControl"(error in=w819, "Image Center Position"=w822) -> ()  [unwired: 1 in, 2 out]
            n292 = String To Path(string=w906) -> (path=w858:path)
            n293 = call "sub_thresh_swing_subvi.vi"("Path"=w858, "NumPts"=w850, "Row Start"=w856) -> ("Index"=w851:dbl, "XY Graph"=w846:cluster{dbl[], dbl[]}[], "Sub Threshold Swing"=w859:dbl)  [unwired: 8 in, 2 out]
            n294 = Decimate 1D Array(w846) -> (w849:cluster{dbl[], dbl[]}[])  [unwired: 1 out]
            n295 = Array To Cluster(array=w849) -> (cluster=w847:T5)
            n296 = Unbundle(w847) -> ("[0]"=w848:cluster{dbl[], dbl[]})  [unwired: 8 out]
            n297 = Unbundle(w848) -> (w845:dbl[], w844:dbl[])
            n298 = local write "Calc: STS"(w859) -> ()
            n299 = local write "XY Graph 2"(w846) -> ()
            n300 = local write "Index 2"(w851) -> ()
            n301 = call "mobility_subvi_07_12a_JW.vi"("Path"=w858, "NumPts"=w857, 11:w856) -> ("Dielectric (d)"=w861:dbl, "Capacitance (C)"=w818:dbl, "Index"=w866:dbl, "XY Graph"=w869:cluster{dbl[], dbl[]}[], "Length"=w860:dbl, "Vt"=w862:dbl, "Width"=w834:dbl, "Table Control"=w904:string[][], "Table Control 2"=w903:string[][], 14:w843, "Mobility"=w902:dbl)  [unwired: 2 in]
            n302 = local write "Rec: Dielectric (d)"(w861) -> ()
            n303 = local write "Calc: VT"(w862) -> ()
            n304 = local write "New Dielectric"(w861) -> ()
            n305 = Decimate 1D Array(w869) -> (w870:cluster{dbl[], dbl[]}[])  [unwired: 1 out]
            n306 = Array To Cluster(array=w870) -> (cluster=w872:T5)
            n307 = local write "Table Control"(w904) -> ()
            n308 = Unbundle(w872) -> ("[0]"=w871:cluster{dbl[], dbl[]})  [unwired: 8 out]
            n309 = Unbundle(w871) -> (w853:dbl[], w852:dbl[])
            n310 = local write "Cal: Mobility-Sat"(w902) -> ()
            n311 = local write "XY Graph"(w869) -> ()
            n312 = local write "Table Control 2"(w903) -> ()
            n313 = Array Subset(array=w853, index=w866, length=w857) -> (w868:dbl[])
            n314 = Array Subset(array=w852, index=w866, length=w857) -> (w867:dbl[])
            n315 = Unbundle(w843) -> (w842, w841, w840, w817, w816, w815, w814)
            n316 = local write "Rec: On/Off"(w840) -> ()
            n317 = local write "Rec: Length"(w860) -> ()
            n318 = local write "Width"(w834) -> ()
            n319 = local write "Array 2"(w867) -> ()
            n320 = local write "Array"(w868) -> ()
            n321 = local write "Slide"(w866) -> ()
            n322 = local write "Index"(w866) -> ()
            n323 = local write "Date Recorded"(w818) -> ()
            n324 = local write "Rec: STS"(w841) -> ()
            n325 = local write "Solvent Recorded"(w816) -> ()
            n326 = local write "Concentration Recorded"(w815) -> ()
            n327 = local write "Method Recorded"(w817) -> ()
            n328 = local write "Rec: VT"(w842) -> ()
            n329 = Array Subset(array=w845, index=w851, length=w850) -> (w855:dbl[])
            n330 = Array Subset(array=w844, index=w851, length=w850) -> (w854:dbl[])
            n331 = local write "New Width"(w834) -> ()
            n332 = local write "Material Recorded"(w814) -> ()
            n333 = local write "Data File"(w858) -> ()
            n334 = local write "New Length"(w860) -> ()
            n335 = local write "Array 8"(w855) -> ()
            n336 = local write "Array 7"(w854) -> ()
            n337 = call-poly <vilib>:"Read From Spreadsheet File.vi"("file path (dialog if empty)"=w858) -> ("all rows"=w891:string[][])  [unwired: 6 in, 4 out]
            n338 = local read "Image Folder"() -> (w825:path)
            n339 = Array Size(array=w891) -> (size(s)=w890:i32[])
            n340 = List Folder(path=w825, error in=w828) -> (filenames=w884:string[], error out=w829:errorcluster)  [unwired: 2 in, 2 out]
            n341 = Index Array(array=w890, index=w889) -> (element=w864:i32)
            n342 = Subtract(x=w864, y=20) -> (x-y=w863:i32)
            n343 = property on="Slide" class="Slide (strict)"("Scale.Maximum"=w863) -> ()  [unwired: 2 in, 2 out]
            n344 = Array Subset(array=w891, index (row)=w889, index (col)=w889, length (col)=3) -> (w892:string[][])  [unwired: 1 in]
            n345 = Reshape Array(w892, w864) -> (w873:string[])
            n346 = local read "No Image"() -> (w835:path)
            n347 = Search 1D Array(1D array=w873, element="Mobility (cm^2/Vs):") -> (index of element=w878:i32)  [unwired: 1 in]
            n348 = Search 1D Array(1D array=w873, element="Index:") -> (index of element=w886:i32)  [unwired: 1 in]
            n349 = Increment(x=w886) -> (x+1=w887:i32)
            n350 = Index Array(array=w873, index=w887) -> (element=w827:string)
            n351 = while {
              tunnel: w884 -> [w921]
              tunnel: w827 -> [w919]
              tunnel: [w918] -> _
              tunnel: [w918] -> w883
              tunnel: w864 -> [w917]
              i -> [w918]
              stop <- w914 stop-if-true
              n352 = Index Array(array=w921, index=w918) -> (element=w922:string)
              n353 = xnode "Match Regular Expression"("input string"=w922, "regular expression"=w919) -> ("whole match"=w920:string)  [unwired: 4 in, 4 out]
              n354 = Equal?(x=w920, y=w919) -> (x = y?=w916:bool)
              n355 = Equal?(x=w917, y=w918) -> (x = y?=w915:bool)
              n356 = Or(x=w916, y=w915) -> (x .or. y?=w914:bool)
            }
            n357 = local write "Index"(w827) -> ()
            n358 = Increment(x=w878) -> (x+1=w877:i32)
            n359 = Build Path(base path=w825, name or relative path="ROI") -> (appended path=w824:path)
            n360 = Index Array(array=w873, index=w877) -> (element=w875:string)
            n361 = Fract/Exp String To Number(string=w875) -> (number=w874:dbl)  [unwired: 3 in, 1 out]
            n362 = local write "Rec: Mobility-Sat"(w874) -> ()
            n363 = Build Path(base path=w824, name or relative path=w827) -> (appended path=w833:path)
            n364 = invoke on="Image Out" class="ImageControl" method="Clear ROI"(error in=w829) -> (error out=w832:errorcluster)  [unwired: 2 in, 2 out]
            n365 = Path To String(path=w825) -> (string=w881:string)
            n366 = call <vilib>:"Check if File or Folder Exists.vi"("error in (no error)"=w832, "path"=w833) -> ("file or folder exists?"=w830:bool, "dup path"=w831:path)  [unwired: 7 in, 1 out]
            n367 = case shown="True" w830 {
              tunnel: w831 -> [_ w909]
              frame False {
              }
              frame True {
                n368 = Read from Text File(file (use dialog)=w909) -> (text=w913:string)  [unwired: 3 in, 3 out]
                n369 = property on="Image Out" class="ImageControl"() -> ("ROI"=w910:T6)  [unwired: 2 in, 2 out]
                n370 = Unflatten From String(type=w910, binary string=w913) -> (value=w911:T6, error out=w912:errorcluster)  [unwired: 3 in, 1 out]
                n371 = property on="Image Out" class="ImageControl"(error in=w912, "ROI"=w911) -> ()  [unwired: 1 in, 2 out]
              }
            }
            n372 = Index Array(array=w884, index=w883) -> (element=w838:string)
            n373 = Empty String/Path?(string/path=w838) -> (empty?=w839:bool)
            n374 = Concatenate Strings(w881, "\\", w838) -> (w880:string)
            n375 = String To Path(string=w880) -> (path=w837:path)
            n376 = Select(t=w835, s=w839, f=w837) -> (s? t:f=w836:path)
            n377 = call "Vision Acquisition4"("Image Path"=w836) -> ("Image Out"=w882:T2)  [unwired: 25 in, 1 out]
            n378 = local write "Image File"(w836) -> ()
            n379 = local write "Image Out 2"(w882) -> ()
            n380 = local write "Image Out"(w882) -> ()
            n381 = invoke on="Image Out" class="ImageControl" method="Clear ROI"() -> ()  [unwired: 3 in, 3 out]
            n382 = local write "Image Name"(w838) -> ()
          }
          event "Data File": Value Change {
            w1108 = 0
            n383 = event-data() -> ()  [unwired: 1 in, 5 out]
            n384 = local read "NumPts"() -> (w1076:dbl)
            n385 = local read "Row Start"() -> (w1075:dbl)
            n386 = local read "Data File"() -> (w1104:path)
            n387 = local read "NumPts 2"() -> (w1069:dbl)
            n388 = property on="Image Out" class="ImageControl"() -> (error out=w1037:errorcluster, "Image Center Position"=w1041:cluster{"X":u32, "Y":u32})  [unwired: 2 in, 1 out]
            n389 = Strip Path(path=w1104) -> (stripped path=w1103:path, name=w1121:string)
            n390 = local write "Data Folder"(w1103) -> ()
            n391 = List Folder(path=w1103) -> (filenames=w1113:string[], error out=w1047:errorcluster)  [unwired: 3 in, 2 out]
            n392 = Unbundle(w1041) -> ("X"=w1039:u32)  [unwired: 1 out]
            n393 = Path To String(path=w1103) -> (string=w1122:string)
            n394 = Search 1D Array(1D array=w1113, element=w1121) -> (index of element=w1114:i32)  [unwired: 1 in]
            n395 = Index Array(array=w1113, index=w1114) -> (element=w1115:string)
            n396 = Bundle("X"=w1039, 0) -> (w1040:cluster{"X":u32, i32})  [unwired: 1 in]
            n397 = local write "Data Name"(w1115) -> ()
            n398 = property on="Image Out" class="ImageControl"(error in=w1037, "Image Center Position"=w1040) -> ()  [unwired: 1 in, 2 out]
            n399 = Concatenate Strings(w1122, "\\", w1115) -> (w1120:string)
            n400 = String To Path(string=w1120) -> (path=w1077:path)
            n401 = call "sub_thresh_swing_subvi.vi"("Path"=w1077, "NumPts"=w1069, "Row Start"=w1075) -> ("Index"=w1070:dbl, "XY Graph"=w1065:cluster{dbl[], dbl[]}[], "Sub Threshold Swing"=w1074:dbl)  [unwired: 8 in, 2 out]
            n402 = Decimate 1D Array(w1065) -> (w1068:cluster{dbl[], dbl[]}[])  [unwired: 1 out]
            n403 = Array To Cluster(array=w1068) -> (cluster=w1066:T5)
            n404 = Unbundle(w1066) -> ("[0]"=w1067:cluster{dbl[], dbl[]})  [unwired: 8 out]
            n405 = Unbundle(w1067) -> (w1063:dbl[], w1062:dbl[])
            n406 = local write "Index 2"(w1070) -> ()
            n407 = call "mobility_subvi_07_12a_JW.vi"("Path"=w1077, "NumPts"=w1076, 11:w1075) -> ("Dielectric (d)"=w1079:dbl, "Index"=w1084:dbl, "XY Graph"=w1087:cluster{dbl[], dbl[]}[], "Length"=w1078:dbl, "Vt"=w1080:dbl, "Width"=w1052:dbl, "Table Control"=w1118:string[][], "Table Control 2"=w1117:string[][], 14:w1059, "Mobility"=w1116:dbl)  [unwired: 2 in, 1 out]
            n408 = local write "Rec: Dielectric (d)"(w1079) -> ()
            n409 = local write "New Dielectric"(w1079) -> ()
            n410 = Decimate 1D Array(w1087) -> (w1088:cluster{dbl[], dbl[]}[])  [unwired: 1 out]
            n411 = local write "Table Control"(w1118) -> ()
            n412 = Array To Cluster(array=w1088) -> (cluster=w1090:T5)
            n413 = Unbundle(w1090) -> ("[0]"=w1089:cluster{dbl[], dbl[]})  [unwired: 8 out]
            n414 = local write "Calc: VT"(w1080) -> ()
            n415 = local write "Calc: STS"(w1074) -> ()
            n416 = local write "Cal: Mobility-Sat"(w1116) -> ()
            n417 = Unbundle(w1089) -> (w1064:dbl[], w1071:dbl[])
            n418 = local write "XY Graph"(w1087) -> ()
            n419 = local write "Rec: Length"(w1078) -> ()
            n420 = local write "Table Control 2"(w1117) -> ()
            n421 = local write "XY Graph 2"(w1065) -> ()
            n422 = Unbundle(w1059) -> ("Vt"=w1061, "STS"=w1060, "On/Off"=w1058)
            n423 = local write "Rec: On/Off"(w1058) -> ()
            n424 = Array Subset(array=w1063, index=w1070, length=w1069) -> (w1073:dbl[])
            n425 = Array Subset(array=w1062, index=w1070, length=w1069) -> (w1072:dbl[])
            n426 = local write "Width"(w1052) -> ()
            n427 = Array Subset(array=w1064, index=w1084, length=w1076) -> (w1086:dbl[])
            n428 = Array Subset(array=w1071, index=w1084, length=w1076) -> (w1085:dbl[])
            n429 = local write "Array 8"(w1073) -> ()
            n430 = local write "Array 7"(w1072) -> ()
            n431 = local write "Rec: STS"(w1060) -> ()
            n432 = local write "Rec: VT"(w1061) -> ()
            n433 = local write "New Length"(w1078) -> ()
            n434 = local write "New Width"(w1052) -> ()
            n435 = local write "Array 2"(w1085) -> ()
            n436 = local write "Array"(w1086) -> ()
            n437 = local write "Data File"(w1077) -> ()
            n438 = local read "Image Folder"() -> (w1043:path)
            n439 = local write "Index"(w1084) -> ()
            n440 = local write "Slide"(w1084) -> ()
            n441 = List Folder(path=w1043, error in=w1047) -> (filenames=w1101:string[], error out=w1046:errorcluster)  [unwired: 2 in, 2 out]
            n442 = call-poly <vilib>:"Read From Spreadsheet File.vi"("file path (dialog if empty)"=w1077) -> ("all rows"=w1110:string[][])  [unwired: 6 in, 4 out]
            n443 = Array Size(array=w1110) -> (size(s)=w1109:i32[])
            n444 = Index Array(array=w1109, index=w1108) -> (element=w1083:i32)
            n445 = Subtract(x=w1083, y=20) -> (x-y=w1081:i32)
            n446 = property on="Slide" class="Slide (strict)"("Scale.Maximum"=w1081) -> ()  [unwired: 2 in, 2 out]
            n447 = Array Subset(array=w1110, index (row)=w1108, index (col)=w1108, length (col)=3) -> (w1111:string[][])  [unwired: 1 in]
            n448 = Reshape Array(w1111, w1083) -> (w1091:string[])
            n449 = Search 1D Array(1D array=w1091, element="Index:") -> (index of element=w1105:i32)  [unwired: 1 in]
            n450 = Increment(x=w1105) -> (x+1=w1106:i32)
            n451 = Index Array(array=w1091, index=w1106) -> (element=w1045:string)
            n452 = while {
              tunnel: w1101 -> [w1135]
              tunnel: w1045 -> [w1133]
              tunnel: [w1132] -> _
              tunnel: [w1132] -> w1100
              tunnel: w1083 -> [w1131]
              i -> [w1132]
              stop <- w1128 stop-if-true
              n453 = Index Array(array=w1135, index=w1132) -> (element=w1136:string)
              n454 = xnode "Match Regular Expression"("input string"=w1136, "regular expression"=w1133) -> ("whole match"=w1134:string)  [unwired: 4 in, 4 out]
              n455 = Equal?(x=w1134, y=w1133) -> (x = y?=w1130:bool)
              n456 = Equal?(x=w1131, y=w1132) -> (x = y?=w1129:bool)
              n457 = Or(x=w1130, y=w1129) -> (x .or. y?=w1128:bool)
            }
            n458 = local write "Index"(w1045) -> ()
            n459 = Search 1D Array(1D array=w1091, element="Mobility (cm^2/Vs):") -> (index of element=w1096:i32)  [unwired: 1 in]
            n460 = Increment(x=w1096) -> (x+1=w1095:i32)
            n461 = Index Array(array=w1091, index=w1095) -> (element=w1093:string)
            n462 = Fract/Exp String To Number(string=w1093) -> (number=w1092:dbl)  [unwired: 3 in, 1 out]
            n463 = local write "Rec: Mobility-Sat"(w1092) -> ()
            n464 = Build Path(base path=w1043, name or relative path="ROI") -> (appended path=w1042:path)
            n465 = Path To String(path=w1043) -> (string=w1099:string)
            n466 = local read "No Image"() -> (w1053:path)
            n467 = Build Path(base path=w1042, name or relative path=w1045) -> (appended path=w1051:path)
            n468 = invoke on="Image Out" class="ImageControl" method="Clear ROI"(error in=w1046) -> (error out=w1050:errorcluster)  [unwired: 2 in, 2 out]
            n469 = Index Array(array=w1101, index=w1100) -> (element=w1056:string)
            n470 = Empty String/Path?(string/path=w1056) -> (empty?=w1057:bool)
            n471 = Concatenate Strings(w1099, "\\", w1056) -> (w1098:string)
            n472 = String To Path(string=w1098) -> (path=w1055:path)
            n473 = Select(t=w1053, s=w1057, f=w1055) -> (s? t:f=w1054:path)
            n474 = call "Vision Acquisition3"("Image Path"=w1054) -> ("Image Out"=w1102:T2)  [unwired: 25 in, 1 out]
            n475 = local write "Image File"(w1054) -> ()
            n476 = local write "Image Out 2"(w1102) -> ()
            n477 = local write "Image Out"(w1102) -> ()
            n478 = local write "Image Name"(w1056) -> ()
            n479 = call <vilib>:"Check if File or Folder Exists.vi"("error in (no error)"=w1050, "path"=w1051) -> ("file or folder exists?"=w1048:bool, "dup path"=w1049:path)  [unwired: 7 in, 1 out]
            n480 = invoke on="Image Out" class="ImageControl" method="Clear ROI"() -> ()  [unwired: 3 in, 3 out]
            n481 = case shown="True" w1048 {
              tunnel: w1049 -> [_ w1123]
              frame False {
              }
              frame True {
                n482 = Read from Text File(file (use dialog)=w1123) -> (text=w1127:string)  [unwired: 3 in, 3 out]
                n483 = property on="Image Out" class="ImageControl"() -> ("ROI"=w1124:T6)  [unwired: 2 in, 2 out]
                n484 = Unflatten From String(type=w1124, binary string=w1127) -> (value=w1125:T6, error out=w1126:errorcluster)  [unwired: 3 in, 1 out]
                n485 = property on="Image Out" class="ImageControl"(error in=w1126, "ROI"=w1125) -> ()  [unwired: 1 in, 2 out]
              }
            }
          }
          event "Up Button": Mouse Down {
            w1320 = 0
            n486 = event-data() -> ()  [unwired: 1 in, 5 out]
            n487 = local read "Row Start"() -> (w1290:dbl)
            n488 = local read "Data File"() -> (w1316:path)
            n489 = local read "NumPts 2"() -> (w1285:dbl)
            n490 = local read "NumPts"() -> (w1291:dbl)
            n491 = property on="Image Out" class="ImageControl"() -> (error out=w1250:errorcluster, "Image Center Position"=w1254:cluster{"X":u32, "Y":u32})  [unwired: 2 in, 1 out]
            n492 = Strip Path(path=w1316) -> (stripped path=w1315:path, name=w1336:string)
            n493 = local write "Data Folder"(w1315) -> ()
            n494 = List Folder(path=w1315) -> (filenames=w1326:string[], error out=w1260:errorcluster)  [unwired: 3 in, 2 out]
            n495 = Path To String(path=w1315) -> (string=w1337:string)
            n496 = Search 1D Array(1D array=w1326, element=w1336) -> (index of element=w1328:i32)  [unwired: 1 in]
            n497 = Equal To 0?(x=w1328) -> (x = 0?=w1329:bool)
            n498 = Unbundle(w1254) -> ("X"=w1252:u32)  [unwired: 1 out]
            n499 = Bundle("X"=w1252, 0) -> (w1253:cluster{"X":u32, i32})  [unwired: 1 in]
            n500 = property on="Image Out" class="ImageControl"(error in=w1250, "Image Center Position"=w1253) -> ()  [unwired: 1 in, 2 out]
            n501 = Array Size(array=w1326) -> (size(s)=w1325:i32)
            n502 = case shown="True" w1329 {
              tunnel: w1328 -> [w1464 _]
              tunnel: [w1463 w1465] -> w1327
              tunnel: w1325 -> [_ w1466]
              frame False {
                n503 = Decrement(x=w1464) -> (x-1=w1463:i32)
              }
              frame True {
                n504 = Decrement(x=w1466) -> (x-1=w1465:i32)
              }
            }
            n505 = Index Array(array=w1326, index=w1327) -> (element=w1330:string)
            n506 = local write "Data Name"(w1330) -> ()
            n507 = Concatenate Strings(w1337, "\\", w1330) -> (w1335:string)
            n508 = String To Path(string=w1335) -> (path=w1292:path)
            n509 = call "sub_thresh_swing_subvi.vi"("Path"=w1292, "NumPts"=w1285, "Row Start"=w1290) -> ("Index"=w1284:dbl, "XY Graph"=w1280:cluster{dbl[], dbl[]}[], "Sub Threshold Swing"=w1293:dbl)  [unwired: 8 in, 2 out]
            n510 = Decimate 1D Array(w1280) -> (w1283:cluster{dbl[], dbl[]}[])  [unwired: 1 out]
            n511 = Array To Cluster(array=w1283) -> (cluster=w1281:T5)
            n512 = Unbundle(w1281) -> ("[0]"=w1282:cluster{dbl[], dbl[]})  [unwired: 8 out]
            n513 = Unbundle(w1282) -> (w1279:dbl[], w1278:dbl[])
            n514 = Array Subset(array=w1278, index=w1284, length=w1285) -> (w1286:dbl[])
            n515 = Array Subset(array=w1279, index=w1284, length=w1285) -> (w1287:dbl[])
            n516 = local write "Calc: STS"(w1293) -> ()
            n517 = local write "Array 8"(w1287) -> ()
            n518 = local write "Array 7"(w1286) -> ()
            n519 = call "mobility_subvi_07_12a_JW.vi"("Path"=w1292, "NumPts"=w1291, 11:w1290) -> ("Dielectric (d)"=w1295:dbl, "Capacitance (C)"=w1249:dbl, "Index"=w1297:dbl, "XY Graph"=w1303:cluster{dbl[], dbl[]}[], "Length"=w1294:dbl, "Vt"=w1296:dbl, "Width"=w1271:dbl, "Table Control"=w1333:string[][], "Table Control 2"=w1332:string[][], 14:w1275, "Mobility"=w1331:dbl)  [unwired: 2 in]
            n520 = local write "Rec: Dielectric (d)"(w1295) -> ()
            n521 = local write "New Dielectric"(w1295) -> ()
            n522 = local write "New Length"(w1294) -> ()
            n523 = local write "New Width"(w1271) -> ()
            n524 = local write "Table Control"(w1333) -> ()
            n525 = Decimate 1D Array(w1303) -> (w1304:cluster{dbl[], dbl[]}[])  [unwired: 1 out]
            n526 = local write "XY Graph 2"(w1280) -> ()
            n527 = local write "Cal: Mobility-Sat"(w1331) -> ()
            n528 = Array To Cluster(array=w1304) -> (cluster=w1306:T5)
            n529 = local write "XY Graph"(w1303) -> ()
            n530 = local write "Rec: Length"(w1294) -> ()
            n531 = local write "Index 2"(w1284) -> ()
            n532 = local write "Table Control 2"(w1332) -> ()
            n533 = Unbundle(w1306) -> ("[0]"=w1305:cluster{dbl[], dbl[]})  [unwired: 8 out]
            n534 = local write "Date Recorded"(w1249) -> ()
            n535 = Unbundle(w1305) -> (w1289:dbl[], w1288:dbl[])
            n536 = local write "Calc: VT"(w1296) -> ()
            n537 = local write "Width"(w1271) -> ()
            n538 = Unbundle(w1275) -> ("Vt"=w1277, "STS"=w1276, "On/Off"=w1274)
            n539 = Array Subset(array=w1289, index=w1297, length=w1291) -> (w1302:dbl[])
            n540 = Array Subset(array=w1288, index=w1297, length=w1291) -> (w1301:dbl[])
            n541 = local write "Data File"(w1292) -> ()
            n542 = local write "Index"(w1297) -> ()
            n543 = local write "Rec: STS"(w1276) -> ()
            n544 = local write "Rec: VT"(w1277) -> ()
            n545 = local write "Rec: On/Off"(w1274) -> ()
            n546 = local write "Array 2"(w1301) -> ()
            n547 = local write "Array"(w1302) -> ()
            n548 = local read "Image Folder"() -> (w1248:path)
            n549 = local write "Slide"(w1297) -> ()
            n550 = List Folder(path=w1248, error in=w1260) -> (filenames=w1314:string[], error out=w1259:errorcluster)  [unwired: 2 in, 2 out]
            n551 = call-poly <vilib>:"Read From Spreadsheet File.vi"("file path (dialog if empty)"=w1292) -> ("all rows"=w1322:string[][])  [unwired: 6 in, 4 out]
            n552 = Array Size(array=w1322) -> (size(s)=w1321:i32[])
            n553 = Index Array(array=w1321, index=w1320) -> (element=w1299:i32)
            n554 = Subtract(x=w1299, y=20) -> (x-y=w1298:i32)
            n555 = property on="Slide" class="Slide (strict)"("Scale.Maximum"=w1298) -> ()  [unwired: 2 in, 2 out]
            n556 = Array Subset(array=w1322, index (row)=w1320, index (col)=w1320, length (col)=3) -> (w1323:string[][])  [unwired: 1 in]
            n557 = Reshape Array(w1323, w1299) -> (w1309:string[])
            n558 = Search 1D Array(1D array=w1309, element="Mobility (cm^2/Vs):") -> (index of element=w1312:i32)  [unwired: 1 in]
            n559 = Increment(x=w1312) -> (x+1=w1311:i32)
            n560 = Index Array(array=w1309, index=w1311) -> (element=w1308:string)
            n561 = Fract/Exp String To Number(string=w1308) -> (number=w1307:dbl)  [unwired: 3 in, 1 out]
            n562 = local write "Rec: Mobility-Sat"(w1307) -> ()
            n563 = Search 1D Array(1D array=w1309, element="Index:") -> (index of element=w1317:i32)  [unwired: 1 in]
            n564 = Increment(x=w1317) -> (x+1=w1318:i32)
            n565 = Index Array(array=w1309, index=w1318) -> (element=w1256:string)
            n566 = while {
              tunnel: w1314 -> [w1350]
              tunnel: w1256 -> [w1348]
              tunnel: [w1347] -> w1313
              tunnel: w1299 -> [w1346]
              i -> [w1347]
              stop <- w1343 stop-if-true
              n567 = Index Array(array=w1350, index=w1347) -> (element=w1351:string)
              n568 = xnode "Match Regular Expression"("input string"=w1351, "regular expression"=w1348) -> ("whole match"=w1349:string)  [unwired: 4 in, 4 out]
              n569 = Equal?(x=w1349, y=w1348) -> (x = y?=w1345:bool)
              n570 = Equal?(x=w1346, y=w1347) -> (x = y?=w1344:bool)
              n571 = Or(x=w1345, y=w1344) -> (x .or. y?=w1343:bool)
            }
            n572 = local write "Index"(w1256) -> ()
            n573 = Build Path(base path=w1248, name or relative path="ROI") -> (appended path=w1257:path)
            n574 = Build Path(base path=w1257, name or relative path=w1256) -> (appended path=w1255:path)
            n575 = invoke on="Image Out" class="ImageControl" method="Clear ROI"(error in=w1259) -> (error out=w1263:errorcluster)  [unwired: 2 in, 2 out]
            n576 = call <vilib>:"Check if File or Folder Exists.vi"("error in (no error)"=w1263, "path"=w1255) -> ("file or folder exists?"=w1261:bool, "dup path"=w1262:path)  [unwired: 7 in, 1 out]
            n577 = local read "No Image"() -> (w1272:path)
            n578 = Index Array(array=w1314, index=w1313) -> (element=w1265:string)
            n579 = Build Path(base path=w1248, name or relative path=w1265) -> (appended path=w1264:path)
            n580 = local write "Image Name"(w1265) -> ()
            n581 = case shown="True" w1261 {
              tunnel: w1262 -> [_ w1338]
              frame False {
              }
              frame True {
                n582 = Read from Text File(file (use dialog)=w1338) -> (text=w1342:string)  [unwired: 3 in, 3 out]
                n583 = property on="Image Out" class="ImageControl"() -> ("ROI"=w1339:T6)  [unwired: 2 in, 2 out]
                n584 = Unflatten From String(type=w1339, binary string=w1342) -> (value=w1340:T6, error out=w1341:errorcluster)  [unwired: 3 in, 1 out]
                n585 = property on="Image Out" class="ImageControl"(error in=w1341, "ROI"=w1340) -> ()  [unwired: 1 in, 2 out]
              }
            }
            n586 = Empty String/Path?(string/path=w1265) -> (empty?=w1273:bool)
            n587 = Select(t=w1272, s=w1273, f=w1264) -> (s? t:f=w1266:path)
            n588 = call "Vision Acquisition5"("Image Path"=w1266) -> ("Image Out"=w1270:T2)  [unwired: 25 in, 1 out]
            n589 = local write "Image File"(w1266) -> ()
            n590 = local write "Image Out 2"(w1270) -> ()
            n591 = local write "Image Out"(w1270) -> ()
            n592 = call <vilib>:"Get File Extension.vi"("file"=w1266) -> ("lowercase file extension"=w1268:string)  [unwired: 7 in, 3 out]
            n593 = local write "String"(w1268) -> ()
            n594 = Search 1D Array(1D array=string[] ["bmp", "jpeg", "png", "jpg", "gif"], element=w1268) -> (index of element=w1267:i32)  [unwired: 1 in]
            n595 = Less Than 0?(x=w1267) -> ()  [unwired: 1 out]
          }
          event "Save Changes? 3": Mouse Down {
            n596 = event-data() -> ()  [unwired: 1 in, 7 out]
            n597 = local read "Image Folder"() -> (w1467:path)
            n598 = Build Path(base path=w1467, name or relative path="ROI") -> (appended path=w1474:path)
            n599 = call <vilib>:"Check if File or Folder Exists.vi"("path"=w1474) -> ("file or folder exists?"=w1476:bool, "dup path"=w1473:path)  [unwired: 8 in, 1 out]
            n600 = case shown="False" w1476 {
              tunnel: w1473 -> [w1478 w1479]
              tunnel: [w1477 w1479] -> w1468
              frame False {
                n601 = Create Folder(path (use dialog)=w1478) -> (created path=w1477:path)  [unwired: 2 in, 2 out]
              }
              frame True {
              }
            }
            n602 = property on="Image Out" class="ImageControl"() -> ("ROI"=w1472:T6)  [unwired: 2 in, 2 out]
            n603 = local read "Index"() -> (w1470:string)
            n604 = Flatten To String(anything=w1472) -> (data string=w1471:string)  [unwired: 3 in, 2 out]
            n605 = Build Path(base path=w1468, name or relative path=w1470) -> (appended path=w1469:path)
            n606 = Write to Text File(file (use dialog)=w1469, text=w1471) -> ()  [unwired: 2 in, 3 out]
          }
          event "Next Button": Mouse Down {
            n607 = event-data() -> ()  [unwired: 1 in, 5 out]
            n608 = local read "XY Graph"() -> (w1492:cluster{dbl[], dbl[]}[])
            n609 = local read "NumPts"() -> (w1493:dbl)
            n610 = local read "Index"() -> (w1494:dbl)
            n611 = Decimate 1D Array(w1492) -> (w1488:cluster{dbl[], dbl[]}[], w1487:cluster{dbl[], dbl[]}[])
            n612 = Array To Cluster(array=w1488) -> (cluster=w1498:T5)
            n613 = Unbundle(w1498) -> ("[0]"=w1497:cluster{dbl[], dbl[]})  [unwired: 8 out]
            n614 = Increment(x=w1494) -> (x+1=w1489:dbl)
            n615 = Unbundle(w1497) -> (w1496:dbl[], w1495:dbl[])
            n616 = Array Subset(array=w1496, index=w1489, length=w1493) -> (w1485:dbl[])
            n617 = local write "Index"(w1489) -> ()
            n618 = Array Subset(array=w1495, index=w1489, length=w1493) -> (w1484:dbl[])
            n619 = Bundle(w1485, w1484) -> (w1491:cluster{dbl[], dbl[]})  [unwired: 1 in]
            n620 = Build Array (concatenate)(w1488, w1487, w1491) -> (w1490:cluster{dbl[], dbl[]}[])
            n621 = local write "XY Graph"(w1490) -> ()
            n622 = local read "New Dielectric"() -> (w1483:dbl)
            n623 = local write "Array 2"(w1484) -> ()
            n624 = local read "New Length"() -> (w1482:dbl)
            n625 = local write "Array"(w1485) -> ()
            n626 = local read "New Width"() -> (w1481:dbl)
            n627 = call "mob_calc_subvi.vi"("Width"=w1481, "Length"=w1482, "Dielectric (d)"=w1483, "Array 2"=w1484, "Array"=w1485) -> ("Vt"=w1480:dbl, "Mobility"=w1486:dbl)  [unwired: 4 in, 1 out]
            n628 = local write "New: Mobility-Sat"(w1486) -> ()
            n629 = local write "New: VT"(w1480) -> ()
          }
          event "Next Button 2": Mouse Down {
            n630 = event-data() -> ()  [unwired: 1 in, 7 out]
            n631 = local read "XY Graph 2"() -> (w1507:cluster{dbl[], dbl[]}[])
            n632 = local read "Index 2"() -> (w1509:dbl)
            n633 = local read "NumPts 2"() -> (w1508:dbl)
            n634 = Decimate 1D Array(w1507) -> (w1503:cluster{dbl[], dbl[]}[], w1502:cluster{dbl[], dbl[]}[])
            n635 = Array To Cluster(array=w1503) -> (cluster=w1513:T5)
            n636 = Unbundle(w1513) -> ("[0]"=w1512:cluster{dbl[], dbl[]})  [unwired: 8 out]
            n637 = Increment(x=w1509) -> (x+1=w1504:dbl)
            n638 = Unbundle(w1512) -> (w1511:dbl[], w1510:dbl[])
            n639 = local write "Index 2"(w1504) -> ()
            n640 = Array Subset(array=w1511, index=w1504, length=w1508) -> (w1500:dbl[])
            n641 = Array Subset(array=w1510, index=w1504, length=w1508) -> (w1499:dbl[])
            n642 = Bundle(w1500, w1499) -> (w1506:cluster{dbl[], dbl[]})  [unwired: 1 in]
            n643 = Build Array (concatenate)(w1503, w1502, w1506) -> (w1505:cluster{dbl[], dbl[]}[])
            n644 = local write "XY Graph 2"(w1505) -> ()
            n645 = local write "Array 8"(w1500) -> ()
            n646 = call "sts_calc_subvi.vi"("Array 2"=w1500, "Array"=w1499) -> ("STS"=w1501:dbl)  [unwired: 9 in]
            n647 = local write "Array 7"(w1499) -> ()
            n648 = local write "New: STS"(w1501) -> ()
          }
          event "Previous Button 2": Mouse Down {
            n649 = event-data() -> ()  [unwired: 1 in, 7 out]
            n650 = local read "XY Graph 2"() -> (w1523:cluster{dbl[], dbl[]}[])
            n651 = local read "NumPts 2"() -> (w1524:dbl)
            n652 = local read "Index 2"() -> (w1516:dbl)
            n653 = Decimate 1D Array(w1523) -> (w1520:cluster{dbl[], dbl[]}[], w1519:cluster{dbl[], dbl[]}[])
            n654 = Array To Cluster(array=w1520) -> (cluster=w1528:T5)
            n655 = Unbundle(w1528) -> ("[0]"=w1527:cluster{dbl[], dbl[]})  [unwired: 8 out]
            n656 = Decrement(x=w1516) -> (x-1=w1517:dbl)
            n657 = Unbundle(w1527) -> (w1526:dbl[], w1525:dbl[])
            n658 = local write "Index 2"(w1517) -> ()
            n659 = Array Subset(array=w1526, index=w1517, length=w1524) -> (w1514:dbl[])
            n660 = Array Subset(array=w1525, index=w1517, length=w1524) -> (w1515:dbl[])
            n661 = Bundle(w1514, w1515) -> (w1522:cluster{dbl[], dbl[]})  [unwired: 1 in]
            n662 = Build Array (concatenate)(w1520, w1519, w1522) -> (w1521:cluster{dbl[], dbl[]}[])
            n663 = local write "XY Graph 2"(w1521) -> ()
            n664 = local write "Array 7"(w1515) -> ()
            n665 = call "sts_calc_subvi.vi"("Array 2"=w1514, "Array"=w1515) -> ("STS"=w1518:dbl)  [unwired: 9 in]
            n666 = local write "Array 8"(w1514) -> ()
            n667 = local write "New: STS"(w1518) -> ()
          }
          event "Previous Button": Mouse Down {
            n668 = event-data() -> ()  [unwired: 1 in, 5 out]
            n669 = local read "XY Graph"() -> (w1542:cluster{dbl[], dbl[]}[])
            n670 = Decimate 1D Array(w1542) -> (w1539:cluster{dbl[], dbl[]}[], w1538:cluster{dbl[], dbl[]}[])
            n671 = local read "NumPts"() -> (w1543:dbl)
            n672 = local read "Index"() -> (w1537:dbl)
            n673 = Array To Cluster(array=w1539) -> (cluster=w1547:T5)
            n674 = Unbundle(w1547) -> ("[0]"=w1546:cluster{dbl[], dbl[]})  [unwired: 8 out]
            n675 = Decrement(x=w1537) -> (x-1=w1536:dbl)
            n676 = Unbundle(w1546) -> (w1545:dbl[], w1544:dbl[])
            n677 = local read "New Dielectric"() -> (w1530:dbl)
            n678 = Array Subset(array=w1545, index=w1536, length=w1543) -> (w1535:dbl[])
            n679 = Array Subset(array=w1544, index=w1536, length=w1543) -> (w1534:dbl[])
            n680 = local write "Index"(w1536) -> ()
            n681 = Bundle(w1535, w1534) -> (w1541:cluster{dbl[], dbl[]})  [unwired: 1 in]
            n682 = Build Array (concatenate)(w1539, w1538, w1541) -> (w1540:cluster{dbl[], dbl[]}[])
            n683 = local write "XY Graph"(w1540) -> ()
            n684 = local read "New Length"() -> (w1531:dbl)
            n685 = local write "Array 2"(w1534) -> ()
            n686 = local read "New Width"() -> (w1532:dbl)
            n687 = call "mob_calc_subvi.vi"("Width"=w1532, "Length"=w1531, "Dielectric (d)"=w1530, "Array 2"=w1534, "Array"=w1535) -> ("Vt"=w1529:dbl, "Mobility"=w1533:dbl)  [unwired: 4 in, 1 out]
            n688 = local write "New: Mobility-Sat"(w1533) -> ()
            n689 = local write "Array"(w1535) -> ()
            n690 = local write "New: VT"(w1529) -> ()
          }
          event "Slide": Value Change {
            n691 = event-data() -> ()  [unwired: 1 in, 5 out]
            n692 = local read "XY Graph"() -> (w1560:cluster{dbl[], dbl[]}[])
            n693 = local read "Slide"() -> (w1549:dbl)
            n694 = Decimate 1D Array(w1560) -> (w1557:cluster{dbl[], dbl[]}[], w1556:cluster{dbl[], dbl[]}[])
            n695 = local read "NumPts"() -> (w1561:dbl)
            n696 = Array To Cluster(array=w1557) -> (cluster=w1565:T5)
            n697 = Unbundle(w1565) -> ("[0]"=w1564:cluster{dbl[], dbl[]})  [unwired: 8 out]
            n698 = Unbundle(w1564) -> (w1563:dbl[], w1562:dbl[])
            n699 = local read "New Dielectric"() -> (w1550:dbl)
            n700 = Array Subset(array=w1563, index=w1549, length=w1561) -> (w1555:dbl[])
            n701 = Array Subset(array=w1562, index=w1549, length=w1561) -> (w1554:dbl[])
            n702 = local write "Index"(w1549) -> ()
            n703 = Bundle(w1555, w1554) -> (w1559:cluster{dbl[], dbl[]})  [unwired: 1 in]
            n704 = Build Array (concatenate)(w1557, w1556, w1559) -> (w1558:cluster{dbl[], dbl[]}[])
            n705 = local write "XY Graph"(w1558) -> ()
            n706 = local read "New Length"() -> (w1551:dbl)
            n707 = local write "Array 2"(w1554) -> ()
            n708 = local read "New Width"() -> (w1552:dbl)
            n709 = call "mob_calc_subvi.vi"("Width"=w1552, "Length"=w1551, "Dielectric (d)"=w1550, "Array 2"=w1554, "Array"=w1555) -> ("Vt"=w1548:dbl, "Mobility"=w1553:dbl)  [unwired: 4 in, 1 out]
            n710 = local write "New: Mobility-Sat"(w1553) -> ()
            n711 = local write "Array"(w1555) -> ()
            n712 = local write "New: VT"(w1548) -> ()
          }
          event "Slide 2": Value Change {
            n713 = event-data() -> ()  [unwired: 1 in, 5 out]
            n714 = local read "XY Graph 2"() -> (w1574:cluster{dbl[], dbl[]}[])
            n715 = local read "Slide 2"() -> (w1569:dbl)
            n716 = Decimate 1D Array(w1574) -> (w1571:cluster{dbl[], dbl[]}[], w1570:cluster{dbl[], dbl[]}[])
            n717 = local read "NumPts 2"() -> (w1575:dbl)
            n718 = Array To Cluster(array=w1571) -> (cluster=w1579:T5)
            n719 = Unbundle(w1579) -> ("[0]"=w1578:cluster{dbl[], dbl[]})  [unwired: 8 out]
            n720 = Unbundle(w1578) -> (w1577:dbl[], w1576:dbl[])
            n721 = Array Subset(array=w1577, index=w1569, length=w1575) -> (w1567:dbl[])
            n722 = Array Subset(array=w1576, index=w1569, length=w1575) -> (w1566:dbl[])
            n723 = local write "Index 2"(w1569) -> ()
            n724 = Bundle(w1567, w1566) -> (w1573:cluster{dbl[], dbl[]})  [unwired: 1 in]
            n725 = Build Array (concatenate)(w1571, w1570, w1573) -> (w1572:cluster{dbl[], dbl[]}[])
            n726 = local write "XY Graph 2"(w1572) -> ()
            n727 = local write "Array 7"(w1566) -> ()
            n728 = local write "Array 8"(w1567) -> ()
            n729 = call "sts_calc_subvi.vi"("Array 2"=w1567, "Array"=w1566) -> ("STS"=w1568:dbl)  [unwired: 9 in]
            n730 = local write "New: STS"(w1568) -> ()
          }
          event "Save Changes?": Mouse Down {
            n731 = event-data() -> ()  [unwired: 1 in, 5 out]
            n732 = flat-sequence {
              tunnel: [w1607] -> w1585
              tunnel: [w1606] -> w1583
              tunnel: [w1606] -> w1582
              tunnel: [w1589] -> w1580
              tunnel: w1585 -> [w1715]
              tunnel: [w1716] -> w1584
              tunnel: w1583 -> [w1716]
              tunnel: w1582 -> [w1714]
              tunnel: [w1712] -> w1581
              tunnel: w1580 -> [w1712]
              tunnel: w1584 -> [w1721]
              tunnel: w1581 -> [w1720]
              frame #0 {
                w1594 = -1
                w1587 = "S.T.S. (V/decade):"
                w1588 = "Threshold V (V):"
                (unwired) 3
                w1592 = 1
                n733 = local read "New: Mobility-Sat"() -> (w1629:dbl)
                n734 = local read "Data File"() -> (w1607:path)
                n735 = local read "New Dielectric"() -> (w1630:dbl)
                n736 = local read "New Width"() -> (w1620:dbl)
                n737 = local read "New Length"() -> (w1618:dbl)
                n738 = flat-sequence {
                  tunnel: [w1643] -> w1586
                  tunnel: w1586 -> [w1660]
                  frame #0 {
                    # "Makes Empty File for Transformer Data"
                    n739 = local read "Data Folder"() -> (w1632:path)
                    n740 = Build Path(base path=w1632, name or relative path="Stats") -> (appended path=w1634:path)
                    n741 = call <vilib>:"Check if File or Folder Exists.vi"("path"=w1634) -> ("file or folder exists?"=w1635:bool, "dup path"=w1636:path)  [unwired: 8 in, 1 out]
                    n742 = case shown="False" w1635 {
                      tunnel: [w1640 w1642] -> w1637
                      tunnel: w1636 -> [w1641 w1642]
                      frame False {
                        n743 = Create Folder(path (use dialog)=w1641) -> (created path=w1640:path)  [unwired: 2 in, 2 out]
                      }
                      frame True {
                      }
                    }
                    n744 = Build Path(base path=w1637, name or relative path="Tranformer Data.txt") -> (appended path=w1639:path)
                    n745 = call-poly <vilib>:"Write To Spreadsheet File.vi"("append to file? (new file:F)"=TRUE, "file path (dialog if empty)"=w1639) -> ()  [unwired: 6 in, 1 out]
                  }
                  frame #1 {
                    # "Adds Headers if they don't exist"
                    n746 = Concatenate Strings("Stats\\", "Tranformer Data.txt") -> (w1650:string)
                    n747 = local read "Data Folder"() -> (w1649:path)
                    n748 = Build Path(base path=w1649, name or relative path=w1650) -> (appended path=w1643:path)
                    n749 = call-poly <vilib>:"Read From Spreadsheet File.vi"("file path (dialog if empty)"=w1643) -> ("first row"=w1648:string[])  [unwired: 6 in, 4 out]
                    n750 = Search 1D Array(1D array=w1648, element="DeviceID") -> (index of element=w1646:i32)  [unwired: 1 in]
                    n751 = Equal?(x=w1646, y=0) -> (x = y?=w1644:bool)
                    n752 = case shown="False" w1644 {
                      tunnel: w1643 -> [w1654 _]
                      frame False {
                        n753 = local read "Transformer \nHeaders"() -> (w1653:string[])
                        n754 = call-poly <vilib>:"Write To Spreadsheet File.vi"("1D data"=w1653, "file path (dialog if empty)"=w1654) -> ()  [unwired: 6 in, 1 out]
                      }
                      frame True {
                      }
                    }
                  }
                  frame #2 {
                    # "Adds current device if it doesn't exist"
                    n755 = local read "Current \nRecord"() -> (w1659:string[])
                    n756 = Index Array(array=w1659, index=0) -> (element=w1658:string)
                    n757 = Concatenate Strings("Stats\\", "Tranformer Data.txt") -> (w1663:string)
                    n758 = local read "Data Folder"() -> (w1662:path)
                    n759 = local write "Current Device ID"(w1658) -> ()
                    n760 = local read "Current Device ID"() -> (w1668:string)
                    n761 = Build Path(base path=w1662, name or relative path=w1663) -> (appended path=w1661:path)
                    n762 = call-poly <vilib>:"Read From Spreadsheet File.vi"("file path (dialog if empty)"=w1661) -> ("all rows"=w1655:string[][])  [unwired: 6 in, 4 out]
                    n763 = Index Array(array=w1655, index (col)=0) -> (element=w1656:string[])  [unwired: 1 in]
                    n764 = Search 1D Array(1D array=w1656, element=w1668) -> (index of element=w1657:i32)  [unwired: 1 in]
                    n765 = Equal?(x=w1657, y=-1) -> (x = y?=w1670:bool)
                    n766 = case shown="False" w1670 {
                      tunnel: w1660 -> [w1673 w1684]
                      tunnel: w1657 -> [w1676 _]
                      tunnel: w1655 -> [w1677 _]
                      frame False {
                        n767 = local read "Current \nRecord"() -> (w1675:string[])
                        n768 = Replace Array Subset(array=w1677, new element=w1675, index (row)=w1676) -> (w1674:string[][])  [unwired: 1 in]
                        n769 = flat-sequence {
                          tunnel: w1673 -> [w1678]
                          tunnel: w1674 -> [w1679]
                          tunnel: [w1679] -> w1672
                          tunnel: [w1678] -> w1671
                          tunnel: w1672 -> [w1681]
                          tunnel: w1671 -> [w1680]
                          frame #0 {
                            n770 = Delete(path (use dialog)=w1678) -> ()  [unwired: 4 in, 3 out]
                          }
                          frame #1 {
                            n771 = call-poly <vilib>:"Write To Spreadsheet File.vi"("append to file? (new file:F)"=TRUE, "2D data"=w1681, "file path (dialog if empty)"=w1680) -> ()  [unwired: 5 in, 1 out]
                          }
                        }
                      }
                      frame True {
                        n772 = local read "Current \nRecord"() -> (w1683:string[])
                        n773 = call-poly <vilib>:"Write To Spreadsheet File.vi"("append to file? (new file:F)"=TRUE, "1D data"=w1683, "file path (dialog if empty)"=w1684) -> ()  [unwired: 5 in, 1 out]
                      }
                    }
                  }
                }
                n774 = call-poly <vilib>:"Read From Spreadsheet File.vi"("file path (dialog if empty)"=w1607) -> ("all rows"=w1599:string[][])  [unwired: 6 in, 4 out]
                n775 = Number To Fractional String(number=w1618) -> (F-format string=w1610:string)  [unwired: 3 in]
                n776 = Replace Array Subset(array=w1599, new element=w1610, index (row)=12, index (col)=w1592) -> (w1614:string[][])
                n777 = Number To Fractional String(number=w1620) -> (F-format string=w1621:string)  [unwired: 3 in]
                n778 = Replace Array Subset(array=w1614, new element=w1621, index (row)=13, index (col)=w1592) -> (w1616:string[][])
                n779 = Number To Fractional String(number=w1629) -> (F-format string=w1608:string)  [unwired: 3 in]
                n780 = Number To Fractional String(number=w1630) -> (F-format string=w1609:string)  [unwired: 3 in]
                n781 = Number To Decimal String(number=w1618) -> (decimal integer string=w1617:string)  [unwired: 1 in]
                n782 = Strip Path(path=w1607) -> (stripped path=w1628:path)  [unwired: 1 out]
                n783 = local read "Index"() -> (w1623:string)
                n784 = Replace Array Subset(array=w1616, new element=w1608, index (row)=15, index (col)=w1592) -> (w1615:string[][])
                n785 = Number To Decimal String(number=w1620) -> (decimal integer string=w1619:string)  [unwired: 1 in]
                n786 = Path To String(path=w1628) -> (string=w1626:string)
                n787 = Replace Array Subset(array=w1615, new element=w1609, index (row)=7, index (col)=w1592) -> (w1591:string[][])
                n788 = call "Build Text"("Index"=w1623, "Length"=w1617, "Width"=w1619) -> ("Result"=w1624:string)  [unwired: 11 in, 1 out]
                n789 = Concatenate Strings(w1626, "\\", w1624) -> (w1625:string)
                n790 = String To Path(string=w1625) -> (path=w1606:path)
                n791 = Array Size(array=w1599) -> (size(s)=w1601:i32[])
                n792 = Index Array(array=w1601, index=0) -> (element=w1600:i32)
                n793 = Array Subset(array=w1599, index (row)=0, index (col)=0) -> (w1605:string[][])  [unwired: 2 in]
                n794 = Reshape Array(w1605, w1600) -> (w1593:string[])
                n795 = Search 1D Array(1D array=w1593, element=w1588) -> (index of element=w1597:i32)  [unwired: 1 in]
                n796 = Search 1D Array(1D array=w1593, element=w1587) -> (index of element=w1598:i32)  [unwired: 1 in]
                n797 = Equal?(x=w1597, y=w1594) -> (x = y?=w1595:bool)
                n798 = Equal?(x=w1598, y=w1594) -> (x = y?=w1596:bool)
                n799 = case shown="True" w1595 {
                  tunnel: w1597 -> [_ _]
                  tunnel: w1591 -> [w1702 w1710]
                  tunnel: [w1701 w1709] -> w1590
                  tunnel: w1588 -> [_ w1708]
                  frame False {
                    n800 = local read "New: VT"() -> (w1704:dbl)
                    n801 = Number To Fractional String(number=w1704) -> (F-format string=w1700:string)  [unwired: 3 in]
                    n802 = Replace Array Subset(array=w1702, new element=w1700, index (row)=17, index (col)=1) -> (w1701:string[][])
                  }
                  frame True {
                    n803 = local read "New: VT"() -> (w1711:dbl)
                    n804 = Number To Fractional String(number=w1711) -> (F-format string=w1707:string)  [unwired: 3 in]
                    n805 = Build Array(w1708, w1707) -> (w1706:string[])
                    n806 = Insert Into Array(array=w1710, index (row)=17, new element=w1706) -> (w1709:string[][])  [unwired: 1 in]
                  }
                }
                n807 = case shown="True" w1596 {
                  tunnel: w1598 -> [_ _]
                  tunnel: w1590 -> [w1689 w1697]
                  tunnel: [w1688 w1696] -> w1589
                  tunnel: w1587 -> [_ w1694]
                  frame False {
                    n808 = local read "New: STS"() -> (w1691:dbl)
                    n809 = Number To Fractional String(number=w1691) -> (F-format string=w1687:string)  [unwired: 3 in]
                    n810 = Replace Array Subset(array=w1689, new element=w1687, index (row)=18, index (col)=1) -> (w1688:string[][])
                  }
                  frame True {
                    n811 = local read "New: STS"() -> (w1698:dbl)
                    n812 = Number To Fractional String(number=w1698) -> (F-format string=w1695:string)  [unwired: 3 in]
                    n813 = Build Array(w1694, w1695) -> (w1693:string[])
                    n814 = Insert Into Array(array=w1697, index (row)=18, new element=w1693) -> (w1696:string[][])  [unwired: 1 in]
                  }
                }
              }
              frame #1 {
                n815 = Equal?(x=w1715, y=w1714) -> (x = y?=w1713:bool)
                n816 = case shown="False" w1713 {
                  tunnel: w1715 -> [w1719 _]
                  tunnel: w1714 -> [w1718 _]
                  frame False {
                    n817 = Move(source path=w1719, 9:TRUE, 10:w1718) -> ()  [unwired: 2 in, 3 out]
                  }
                  frame True {
                  }
                }
              }
              frame #2 {
                n818 = local write "Data File"(w1721) -> ()
                n819 = call-poly <vilib>:"Write To Spreadsheet File.vi"("2D data"=w1720, "file path (dialog if empty)"=w1721) -> ()  [unwired: 6 in, 1 out]
              }
            }
          }
          event "Save Changes? 2": Mouse Down {
            n820 = event-data() -> ()  [unwired: 1 in, 5 out]
            n821 = stacked-sequence {
              seq-local: [w1798 _ _ _ _] -> [_ w1851 _ _ _]
              seq-local: [w1797 _ _ _ _] -> [_ w1852 _ _ _]
              seq-local: [w1797 _ _ _ _] -> [_ w1850 _ _ _]
              seq-local: [w1780 _ _ _ _] -> [_ w1848 _ _ _]
              seq-local: [_ w1852 _ _ _] -> [_ _ w1857 _ _]
              seq-local: [_ w1848 _ _ _] -> [_ _ w1856 _ _]
              frame #0 {
                w1785 = -1
                w1778 = "S.T.S. (V/decade):"
                w1779 = "Threshold V (V):"
                (unwired) 3
                w1783 = 1
                n822 = local read "Data File"() -> (w1798:path)
                n823 = local read "New Width"() -> (w1811:dbl)
                n824 = local read "New Dielectric"() -> (w1821:dbl)
                n825 = local read "New Length"() -> (w1809:dbl)
                n826 = local read "New: Mobility-Sat"() -> (w1820:dbl)
                n827 = call-poly <vilib>:"Read From Spreadsheet File.vi"("file path (dialog if empty)"=w1798) -> ("all rows"=w1790:string[][])  [unwired: 6 in, 4 out]
                n828 = Number To Fractional String(number=w1809) -> (F-format string=w1801:string)  [unwired: 3 in]
                n829 = Replace Array Subset(array=w1790, new element=w1801, index (row)=12, index (col)=w1783) -> (w1805:string[][])
                n830 = Number To Fractional String(number=w1811) -> (F-format string=w1812:string)  [unwired: 3 in]
                n831 = Replace Array Subset(array=w1805, new element=w1812, index (row)=13, index (col)=w1783) -> (w1807:string[][])
                n832 = Number To Fractional String(number=w1820) -> (F-format string=w1799:string)  [unwired: 3 in]
                n833 = Number To Fractional String(number=w1821) -> (F-format string=w1800:string)  [unwired: 3 in]
                n834 = Number To Decimal String(number=w1809) -> (decimal integer string=w1808:string)  [unwired: 1 in]
                n835 = Strip Path(path=w1798) -> (stripped path=w1819:path)  [unwired: 1 out]
                n836 = local read "Index"() -> (w1814:string)
                n837 = Replace Array Subset(array=w1807, new element=w1799, index (row)=15, index (col)=w1783) -> (w1806:string[][])
                n838 = Number To Decimal String(number=w1811) -> (decimal integer string=w1810:string)  [unwired: 1 in]
                n839 = Path To String(path=w1819) -> (string=w1817:string)
                n840 = Replace Array Subset(array=w1806, new element=w1800, index (row)=7, index (col)=w1783) -> (w1782:string[][])
                n841 = call "Build Text2"("Index"=w1814, "Length"=w1808, "Width"=w1810) -> ("Result"=w1815:string)  [unwired: 11 in, 1 out]
                n842 = Concatenate Strings(w1817, "\\", w1815) -> (w1816:string)
                n843 = String To Path(string=w1816) -> (path=w1797:path)
                n844 = Array Size(array=w1790) -> (size(s)=w1792:i32[])
                n845 = Index Array(array=w1792, index=0) -> (element=w1791:i32)
                n846 = Array Subset(array=w1790, index (row)=0, index (col)=0) -> (w1796:string[][])  [unwired: 2 in]
                n847 = Reshape Array(w1796, w1791) -> (w1784:string[])
                n848 = Search 1D Array(1D array=w1784, element=w1779) -> (index of element=w1788:i32)  [unwired: 1 in]
                n849 = Search 1D Array(1D array=w1784, element=w1778) -> (index of element=w1789:i32)  [unwired: 1 in]
                n850 = Equal?(x=w1788, y=w1785) -> (x = y?=w1786:bool)
                n851 = Equal?(x=w1789, y=w1785) -> (x = y?=w1787:bool)
                n852 = case shown="True" w1786 {
                  tunnel: w1788 -> [_ _]
                  tunnel: w1782 -> [w1838 w1846]
                  tunnel: [w1837 w1845] -> w1781
                  tunnel: w1779 -> [_ w1844]
                  frame False {
                    n853 = local read "New: VT"() -> (w1840:dbl)
                    n854 = Number To Fractional String(number=w1840) -> (F-format string=w1836:string)  [unwired: 3 in]
                    n855 = Replace Array Subset(array=w1838, new element=w1836, index (row)=17, index (col)=1) -> (w1837:string[][])
                  }
                  frame True {
                    n856 = local read "New: VT"() -> (w1847:dbl)
                    n857 = Number To Fractional String(number=w1847) -> (F-format string=w1843:string)  [unwired: 3 in]
                    n858 = Build Array(w1844, w1843) -> (w1842:string[])
                    n859 = Insert Into Array(array=w1846, index (row)=17, new element=w1842) -> (w1845:string[][])  [unwired: 1 in]
                  }
                }
                n860 = case shown="True" w1787 {
                  tunnel: w1789 -> [_ _]
                  tunnel: w1781 -> [w1825 w1833]
                  tunnel: [w1824 w1832] -> w1780
                  tunnel: w1778 -> [_ w1830]
                  frame False {
                    n861 = local read "New: STS"() -> (w1827:dbl)
                    n862 = Number To Fractional String(number=w1827) -> (F-format string=w1823:string)  [unwired: 3 in]
                    n863 = Replace Array Subset(array=w1825, new element=w1823, index (row)=18, index (col)=1) -> (w1824:string[][])
                  }
                  frame True {
                    n864 = local read "New: STS"() -> (w1834:dbl)
                    n865 = Number To Fractional String(number=w1834) -> (F-format string=w1831:string)  [unwired: 3 in]
                    n866 = Build Array(w1830, w1831) -> (w1829:string[])
                    n867 = Insert Into Array(array=w1833, index (row)=18, new element=w1829) -> (w1832:string[][])  [unwired: 1 in]
                  }
                }
              }
              frame #1 {
                n868 = Equal?(x=w1851, y=w1850) -> (x = y?=w1849:bool)
                n869 = case shown="False" w1849 {
                  tunnel: w1851 -> [w1855 _]
                  tunnel: w1850 -> [w1854 _]
                  frame False {
                    n870 = Move(source path=w1855, 9:TRUE, 10:w1854) -> ()  [unwired: 2 in, 3 out]
                  }
                  frame True {
                  }
                }
              }
              frame #2 {
                n871 = local write "Data File"(w1857) -> ()
                n872 = call-poly <vilib>:"Write To Spreadsheet File.vi"("2D data"=w1856, "file path (dialog if empty)"=w1857) -> ()  [unwired: 6 in, 1 out]
              }
              frame #3 {
                w1921 = 0
                n873 = local read "NumPts 2"() -> (w1880:dbl)
                n874 = local read "NumPts"() -> (w1887:dbl)
                n875 = local read "Row Start"() -> (w1886:dbl)
                n876 = local read "Data File"() -> (w1926:path)
                n877 = property on="Image Out" class="ImageControl"() -> (error out=w1861:errorcluster, "Image Center Position"=w1865:cluster{"X":u32, "Y":u32})  [unwired: 2 in, 1 out]
                n878 = Strip Path(path=w1926) -> (stripped path=w1917:path, name=w1939:string)
                n879 = local write "Data Folder"(w1917) -> ()
                n880 = List Folder(path=w1917) -> (filenames=w1932:string[])  [unwired: 3 in, 3 out]
                n881 = Unbundle(w1865) -> ("X"=w1863:u32)  [unwired: 1 out]
                n882 = Array Size(array=w1932) -> (size(s)=w1927:i32)
                n883 = Path To String(path=w1917) -> (string=w1940:string)
                n884 = Search 1D Array(1D array=w1932, element=w1939) -> (index of element=w1929:i32)  [unwired: 1 in]
                n885 = Bundle("X"=w1863, 0) -> (w1864:cluster{"X":u32, i32})  [unwired: 1 in]
                n886 = Decrement(x=w1927) -> (x-1=w1930:i32)
                n887 = Equal?(x=w1929, y=w1930) -> (x = y?=w1931:bool)
                n888 = case shown="False" w1931 {
                  tunnel: w1929 -> [w2062 _]
                  tunnel: [w2061 0] -> w1928
                  frame False {
                    n889 = Increment(x=w2062) -> (x+1=w2061:i32)
                  }
                  frame True {
                  }
                }
                n890 = Index Array(array=w1932, index=w1928) -> (element=w1933:string)
                n891 = local write "Data Name"(w1933) -> ()
                n892 = Concatenate Strings(w1940, "\\", w1933) -> (w1938:string)
                n893 = property on="Image Out" class="ImageControl"(error in=w1861, "Image Center Position"=w1864) -> ()  [unwired: 1 in, 2 out]
                n894 = String To Path(string=w1938) -> (path=w1888:path)
                n895 = call "sub_thresh_swing_subvi.vi"("Path"=w1888, "NumPts"=w1880, "Row Start"=w1886) -> ("Index"=w1881:dbl, "XY Graph"=w1876:cluster{dbl[], dbl[]}[], "Sub Threshold Swing"=w1889:dbl)  [unwired: 8 in, 2 out]
                n896 = Decimate 1D Array(w1876) -> (w1879:cluster{dbl[], dbl[]}[])  [unwired: 1 out]
                n897 = Array To Cluster(array=w1879) -> (cluster=w1877:T5)
                n898 = Unbundle(w1877) -> ("[0]"=w1878:cluster{dbl[], dbl[]})  [unwired: 8 out]
                n899 = Unbundle(w1878) -> (w1875:dbl[], w1874:dbl[])
                n900 = local write "Calc: STS"(w1889) -> ()
                n901 = local write "XY Graph 2"(w1876) -> ()
                n902 = local write "Index 2"(w1881) -> ()
                n903 = call "mobility_subvi_07_12a_JW.vi"("Path"=w1888, "NumPts"=w1887, 11:w1886) -> ("Dielectric (d)"=w1892:dbl, "Index"=w1897:dbl, "XY Graph"=w1900:cluster{dbl[], dbl[]}[], "Length"=w1890:dbl, "Vt"=w1893:dbl, "Width"=w1891:dbl, "Table Control"=w1936:string[][], "Table Control 2"=w1935:string[][], 14:w1873, "Mobility"=w1934:dbl)  [unwired: 2 in, 1 out]
                n904 = local write "Rec: Dielectric (d)"(w1892) -> ()
                n905 = local write "Calc: VT"(w1893) -> ()
                n906 = local write "New Dielectric"(w1892) -> ()
                n907 = Decimate 1D Array(w1900) -> (w1901:cluster{dbl[], dbl[]}[])  [unwired: 1 out]
                n908 = Array To Cluster(array=w1901) -> (cluster=w1903:T5)
                n909 = local write "Table Control"(w1936) -> ()
                n910 = Unbundle(w1903) -> ("[0]"=w1902:cluster{dbl[], dbl[]})  [unwired: 8 out]
                n911 = Unbundle(w1902) -> (w1883:dbl[], w1882:dbl[])
                n912 = local write "Cal: Mobility-Sat"(w1934) -> ()
                n913 = local write "XY Graph"(w1900) -> ()
                n914 = local write "Table Control 2"(w1935) -> ()
                n915 = Array Subset(array=w1883, index=w1897, length=w1887) -> (w1899:dbl[])
                n916 = Array Subset(array=w1882, index=w1897, length=w1887) -> (w1898:dbl[])
                n917 = local write "Rec: Length"(w1890) -> ()
                n918 = local write "Width"(w1891) -> ()
                n919 = local write "Array 2"(w1898) -> ()
                n920 = Unbundle(w1873) -> ("Vt"=w1872, "STS"=w1871, "On/Off"=w1870)
                n921 = local write "Rec: On/Off"(w1870) -> ()
                n922 = local write "Array"(w1899) -> ()
                n923 = local write "Slide"(w1897) -> ()
                n924 = local write "Index"(w1897) -> ()
                n925 = local write "Rec: STS"(w1871) -> ()
                n926 = local write "Rec: VT"(w1872) -> ()
                n927 = Array Subset(array=w1875, index=w1881, length=w1880) -> (w1885:dbl[])
                n928 = Array Subset(array=w1874, index=w1881, length=w1880) -> (w1884:dbl[])
                n929 = local write "New Width"(w1891) -> ()
                n930 = local write "Data File"(w1888) -> ()
                n931 = local write "New Length"(w1890) -> ()
                n932 = local write "Array 8"(w1885) -> ()
                n933 = local write "Array 7"(w1884) -> ()
                n934 = call-poly <vilib>:"Read From Spreadsheet File.vi"("file path (dialog if empty)"=w1888) -> ("all rows"=w1923:string[][])  [unwired: 6 in, 4 out]
                n935 = local read "Image Folder"() -> (w1911:path)
                n936 = Array Size(array=w1923) -> (size(s)=w1922:i32[])
                n937 = List Folder(path=w1911) -> (filenames=w1916:string[])  [unwired: 3 in, 3 out]
                n938 = Index Array(array=w1922, index=w1921) -> (element=w1895:i32)
                n939 = Subtract(x=w1895, y=20) -> (x-y=w1894:i32)
                n940 = property on="Slide" class="Slide (strict)"("Scale.Maximum"=w1894) -> ()  [unwired: 2 in, 2 out]
                n941 = Array Subset(array=w1923, index (row)=w1921, index (col)=w1921, length (col)=3) -> (w1924:string[][])  [unwired: 1 in]
                n942 = Reshape Array(w1924, w1895) -> (w1904:string[])
                n943 = Search 1D Array(1D array=w1904, element="Mobility (cm^2/Vs):") -> (index of element=w1909:i32)  [unwired: 1 in]
                n944 = Search 1D Array(1D array=w1904, element="Index:") -> (index of element=w1918:i32)  [unwired: 1 in]
                n945 = Increment(x=w1918) -> (x+1=w1919:i32)
                n946 = Index Array(array=w1904, index=w1919) -> (element=w1914:string)
                n947 = while {
                  tunnel: w1916 -> [w1948]
                  tunnel: w1914 -> [w1946]
                  tunnel: [w1945] -> _
                  tunnel: [w1945] -> w1915
                  tunnel: w1895 -> [w1944]
                  i -> [w1945]
                  stop <- w1941 stop-if-true
                  n948 = Index Array(array=w1948, index=w1945) -> (element=w1949:string)
                  n949 = xnode "Match Regular Expression"("input string"=w1949, "regular expression"=w1946) -> ("whole match"=w1947:string)  [unwired: 4 in, 4 out]
                  n950 = Equal?(x=w1947, y=w1946) -> (x = y?=w1943:bool)
                  n951 = Equal?(x=w1944, y=w1945) -> (x = y?=w1942:bool)
                  n952 = Or(x=w1943, y=w1942) -> (x .or. y?=w1941:bool)
                }
                n953 = local write "Index"(w1914) -> ()
                n954 = Increment(x=w1909) -> (x+1=w1908:i32)
                n955 = local read "No Image"() -> (w1866:path)
                n956 = Index Array(array=w1904, index=w1908) -> (element=w1906:string)
                n957 = Fract/Exp String To Number(string=w1906) -> (number=w1905:dbl)  [unwired: 3 in, 1 out]
                n958 = local write "Rec: Mobility-Sat"(w1905) -> ()
                n959 = Path To String(path=w1911) -> (string=w1913:string)
                n960 = local read "Image Out"() -> (w1858:T2)
                n961 = Index Array(array=w1916, index=w1915) -> (element=w1868:string)
                n962 = Empty String/Path?(string/path=w1868) -> (empty?=w1869:bool)
                n963 = Concatenate Strings(w1913, "\\", w1868) -> (w1912:string)
                n964 = local write "Image Name"(w1868) -> ()
                n965 = String To Path(string=w1912) -> (path=w1867:path)
                n966 = Select(t=w1866, s=w1869, f=w1867) -> (s? t:f=w1860:path)
                n967 = local write "Image File"(w1860) -> ()
                n968 = call "IMAQ ReadFile"("File Path"=w1860, "Image"=w1858) -> ("Image Out"=w1859:T2)  [unwired: 5 in, 4 out]
                n969 = local write "Image Out 2"(w1859) -> ()
                n970 = local write "Image Out"(w1859) -> ()
                n971 = invoke on="Image Out" class="ImageControl" method="Clear ROI"() -> ()  [unwired: 3 in, 3 out]
              }
              frame #4 {
                n972 = local read "Image Folder"() -> (w2064:path)
                n973 = Build Path(base path=w2064, name or relative path="ROI") -> (appended path=w2066:path)
                n974 = local read "Index"() -> (w2065:string)
                n975 = Build Path(base path=w2066, name or relative path=w2065) -> (appended path=w2071:path)
                n976 = invoke on="Image Out" class="ImageControl" method="Clear ROI"() -> (error out=w2070:errorcluster)  [unwired: 3 in, 2 out]
                n977 = call <vilib>:"Check if File or Folder Exists.vi"("error in (no error)"=w2070, "path"=w2071) -> ("file or folder exists?"=w2068:bool, "dup path"=w2069:path)  [unwired: 7 in, 1 out]
                n978 = case shown="True" w2068 {
                  tunnel: w2069 -> [_ w2072]
                  frame False {
                  }
                  frame True {
                    n979 = Read from Text File(file (use dialog)=w2072) -> (text=w2076:string)  [unwired: 3 in, 3 out]
                    n980 = property on="Image Out" class="ImageControl"() -> ("ROI"=w2073:T6)  [unwired: 2 in, 2 out]
                    n981 = Unflatten From String(type=w2073, binary string=w2076) -> (value=w2074:T6, error out=w2075:errorcluster)  [unwired: 3 in, 1 out]
                    n982 = property on="Image Out" class="ImageControl"(error in=w2075, "ROI"=w2074) -> ()  [unwired: 1 in, 2 out]
                  }
                }
              }
            }
            n983 = flat-sequence {
              tunnel: [w1735] -> w1722
              tunnel: w1722 -> [w1749]
              frame #0 {
                # "Makes Empty File for Transformer Data"
                n984 = local read "Data Folder"() -> (w1724:path)
                n985 = Build Path(base path=w1724, name or relative path="Stats") -> (appended path=w1726:path)
                n986 = call <vilib>:"Check if File or Folder Exists.vi"("path"=w1726) -> ("file or folder exists?"=w1727:bool, "dup path"=w1728:path)  [unwired: 8 in, 1 out]
                n987 = case shown="False" w1727 {
                  tunnel: [w1732 w1734] -> w1729
                  tunnel: w1728 -> [w1733 w1734]
                  frame False {
                    n988 = Create Folder(path (use dialog)=w1733) -> (created path=w1732:path)  [unwired: 2 in, 2 out]
                  }
                  frame True {
                  }
                }
                n989 = Build Path(base path=w1729, name or relative path="Tranformer Data.txt") -> (appended path=w1731:path)
                n990 = call-poly <vilib>:"Write To Spreadsheet File.vi"("append to file? (new file:F)"=TRUE, "file path (dialog if empty)"=w1731) -> ()  [unwired: 6 in, 1 out]
              }
              frame #1 {
                # "Adds Headers if they don't exist"
                n991 = Concatenate Strings("Stats\\", "Tranformer Data.txt") -> (w1742:string)
                n992 = local read "Data Folder"() -> (w1741:path)
                n993 = Build Path(base path=w1741, name or relative path=w1742) -> (appended path=w1735:path)
                n994 = call-poly <vilib>:"Read From Spreadsheet File.vi"("file path (dialog if empty)"=w1735) -> ("first row"=w1740:string[])  [unwired: 6 in, 4 out]
                n995 = Search 1D Array(1D array=w1740, element="DeviceID") -> (index of element=w1738:i32)  [unwired: 1 in]
                n996 = Equal?(x=w1738, y=0) -> (x = y?=w1736:bool)
                n997 = case shown="False" w1736 {
                  tunnel: w1735 -> [w1746 _]
                  frame False {
                    n998 = local read "Transformer \nHeaders"() -> (w1745:string[])
                    n999 = call-poly <vilib>:"Write To Spreadsheet File.vi"("1D data"=w1745, "file path (dialog if empty)"=w1746) -> ()  [unwired: 6 in, 1 out]
                  }
                  frame True {
                  }
                }
              }
              frame #2 {
                # "Adds current device if it doesn't exist"
                n1000 = local read "Current \nRecord"() -> (w1752:string[])
                n1001 = Index Array(array=w1752, index=0) -> (element=w1751:string)
                n1002 = Concatenate Strings("Stats\\", "Tranformer Data.txt") -> (w1755:string)
                n1003 = local read "Data Folder"() -> (w1754:path)
                n1004 = local write "Current Device ID"(w1751) -> ()
                n1005 = local read "Current Device ID"() -> (w1761:string)
                n1006 = Build Path(base path=w1754, name or relative path=w1755) -> (appended path=w1753:path)
                n1007 = call-poly <vilib>:"Read From Spreadsheet File.vi"("file path (dialog if empty)"=w1753) -> ("all rows"=w1748:string[][])  [unwired: 6 in, 4 out]
                n1008 = Index Array(array=w1748, index (col)=0) -> (element=w1759:string[])  [unwired: 1 in]
                n1009 = Search 1D Array(1D array=w1759, element=w1761) -> (index of element=w1747:i32)  [unwired: 1 in]
                n1010 = Equal?(x=w1747, y=-1) -> (x = y?=w1750:bool)
                n1011 = case shown="False" w1750 {
                  tunnel: w1749 -> [w1763 w1776]
                  tunnel: w1747 -> [w1768 _]
                  tunnel: w1748 -> [w1769 _]
                  frame False {
                    n1012 = local read "Current \nRecord"() -> (w1767:string[])
                    n1013 = Replace Array Subset(array=w1769, new element=w1767, index (row)=w1768) -> (w1764:string[][])  [unwired: 1 in]
                    n1014 = flat-sequence {
                      tunnel: [w1770] -> _
                      tunnel: [w1771] -> _
                      tunnel: [w1771] -> w1766
                      tunnel: [w1770] -> w1765
                      tunnel: w1764 -> [w1771]
                      tunnel: w1763 -> [w1770]
                      tunnel: w1766 -> [w1773]
                      tunnel: w1765 -> [w1772]
                      frame #0 {
                        n1015 = Delete(path (use dialog)=w1770) -> ()  [unwired: 4 in, 3 out]
                      }
                      frame #1 {
                        n1016 = call-poly <vilib>:"Write To Spreadsheet File.vi"("append to file? (new file:F)"=TRUE, "2D data"=w1773, "file path (dialog if empty)"=w1772) -> ()  [unwired: 5 in, 1 out]
                      }
                    }
                  }
                  frame True {
                    n1017 = local read "Current \nRecord"() -> (w1775:string[])
                    n1018 = call-poly <vilib>:"Write To Spreadsheet File.vi"("append to file? (new file:F)"=TRUE, "1D data"=w1775, "file path (dialog if empty)"=w1776) -> ()  [unwired: 5 in, 1 out]
                  }
                }
              }
            }
          }
          event "Export": Mouse Down {
            n1019 = event-data() -> ()  [unwired: 1 in, 7 out]
            n1020 = call "OA_ConnectToOrigin.vi"() -> ("error out"=w2098:errorcluster, "Origin.IOApplication"=w2099:refnum<k7>)  [unwired: 8 in]
            n1021 = local read "Data Folder"() -> (w2077:path)
            n1022 = local read "Project"() -> (w2097:path)
            n1023 = call "OA_Load.vi"("error in (no error)"=w2098, "Path"=w2097, "Origin.IOApplication"=w2099) -> ("error out"=w2090:errorcluster, "Origin.IOApplication"=w2091:refnum<k7>)  [unwired: 1 out]
            n1024 = call "OAExecute.vi"("script"="document -m 3;", "Error IO"=w2090, "Origin.IOApplication"=w2091) -> ("Error IO Out"=w2088:errorcluster, "Origin.IOApplication"=w2089:refnum<k7>)  [unwired: 1 in, 1 out]
            n1025 = Build Path(base path=w2077, name or relative path="Stats") -> (appended path=w2078:path)
            n1026 = flat-sequence {
              tunnel: w2077 -> [w2119]
              tunnel: w2096 -> [w2118]
              tunnel: [w2108] -> w2101
              tunnel: [w2109] -> w2100
              tunnel: w2089 -> [w2113]
              tunnel: w2088 -> [w2112]
              tunnel: w2077 -> [w2135]
              tunnel: w2096 -> [w2134]
              tunnel: w2101 -> [w2130]
              tunnel: w2100 -> [w2131]
              tunnel: [w2125] -> w2095
              tunnel: [w2124] -> w2094
              tunnel: w2077 -> [w2146]
              tunnel: w2096 -> [w2145]
              tunnel: w2095 -> [w2141]
              tunnel: w2094 -> [w2140]
              tunnel: [w2139] -> w2093
              tunnel: [w2138] -> w2092
              tunnel: w2077 -> [w2161]
              tunnel: w2096 -> [w2160]
              tunnel: w2093 -> [w2155]
              tunnel: w2092 -> [w2154]
              tunnel: [w2152] -> w2086
              tunnel: [w2151] -> w2085
              frame #0 {
                n1027 = call "Param_Analysis.vi"("error in (no error)"=w2112, "Folder 2"=w2119, "Parameter String"="Mobility (cm^2/Vs):", "Parameter Name"="Mobility", "Folder"=w2118) -> ("error out"=w2115:errorcluster, "Array 4"=w2105:string[], "Array 3"=w2114:string[][])  [unwired: 3 in, 1 out]
                n1028 = call "Origin_Export.vi"("String 3"="[MobHistTab]Sheet1", "error in (no error)"=w2115, "Array"=w2114, "String 2"="[MOBvsLTable]Mobilities", "String"="pe_cd \"Mobility Chart\";", "Origin.IOApplication"=w2113, "Array 2"=w2105) -> ("reference out"=w2111:refnum<k7>, "error out"=w2110:errorcluster)  [unwired: 2 in, 1 out]
                n1029 = call "OAExecute.vi"("script"="window -a MOBvsLTable;\nwindow -s TV;", "Error IO"=w2110, "Origin.IOApplication"=w2111) -> ("Error IO Out"=w2108:errorcluster, "Origin.IOApplication"=w2109:refnum<k7>)  [unwired: 1 in, 1 out]
              }
              frame #1 {
                n1030 = call "Param_Analysis.vi"("error in (no error)"=w2130, "Folder 2"=w2135, "Parameter String"="On/Off Current:", "Parameter Name"="On_Off_Current", "Folder"=w2134) -> ("error out"=w2129:errorcluster, "Array 4"=w2123:string[], "Array 3"=w2126:string[][])  [unwired: 3 in, 1 out]
                n1031 = call "Origin_Export.vi"("String 3"="[OnOffHistTab]Sheet1", "error in (no error)"=w2129, "Array"=w2126, "String 2"="[OnOffTable]On/Off Ratios", "String"="pe_cd \"OnOff vs L\";", "Origin.IOApplication"=w2131, "Array 2"=w2123) -> ("reference out"=w2125:refnum<k7>, "error out"=w2124:errorcluster)  [unwired: 2 in, 1 out]
              }
              frame #2 {
                n1032 = call "Param_Analysis.vi"("Folder 2"=w2146, "Parameter String"="S.T.S. (V/decade):", "Parameter Name"="STS", "Folder"=w2145) -> ("Array 4"=w2137:string[], "Array 3"=w2142:string[][])  [unwired: 4 in, 2 out]
                n1033 = call "Origin_Export.vi"("String 3"="[SHistTab]Sheet1", "error in (no error)"=w2140, "Array"=w2142, "String 2"="[STable]Threshold Swing", "String"="pe_cd \"Threshold Swing vs L\";", "Origin.IOApplication"=w2141, "Array 2"=w2137) -> ("reference out"=w2138:refnum<k7>, "error out"=w2139:errorcluster)  [unwired: 2 in, 1 out]
              }
              frame #3 {
                n1034 = call "Param_Analysis.vi"("Folder 2"=w2161, "Parameter String"="Threshold V (V):", "Parameter Name"="Threshold_V", "Folder"=w2160) -> ("Array 4"=w2150:string[], "Array 3"=w2153:string[][])  [unwired: 4 in, 2 out]
                n1035 = call "Origin_Export.vi"("String 3"="[VtHistTab]Sheet1", "error in (no error)"=w2155, "Array"=w2153, "String 2"="[VtTable]Threshold Voltages", "String"="pe_cd \"Threshold Voltage vs L\";", "Origin.IOApplication"=w2154, "Array 2"=w2150) -> ("reference out"=w2152:refnum<k7>, "error out"=w2151:errorcluster)  [unwired: 2 in, 1 out]
              }
            }
            n1036 = call <vilib>:"Check if File or Folder Exists.vi"("path"=w2078) -> ("file or folder exists?"=w2103:bool, "dup path"=w2102:path)  [unwired: 8 in, 1 out]
            n1037 = case shown="False" w2103 {
              tunnel: w2102 -> [w2163 w2164]
              tunnel: [w2162 w2164] -> w2096
              frame False {
                n1038 = Create Folder(path (use dialog)=w2163) -> (created path=w2162:path)  [unwired: 2 in, 2 out]
              }
              frame True {
              }
            }
            n1039 = call "File Dialog"("start path"=w2078) -> ("selected path"=w2081:path)  [unwired: 11 in, 3 out]
            n1040 = Path To String(path=w2081) -> (string=w2080:string)
            n1041 = call "OAExecute.vi"("script"="pe_cd /;\npe_cd \"Mobility Chart\"; ", "Error IO"=w2085, "Origin.IOApplication"=w2086) -> ("Error IO Out"=w2082:errorcluster, "Origin.IOApplication"=w2083:refnum<k7>)  [unwired: 1 in, 1 out]
            n1042 = call "OASaveProject.vi"("path"=w2080, "Error IO"=w2082, "Origin.IOApplication"=w2083) -> ()  [unwired: 3 out]
          }
          event "Blank Button": Mouse Down {
            n1043 = event-data() -> ()  [unwired: 1 in, 7 out]
            n1044 = local read "Data File"() -> (w2172:path)
            n1045 = Strip Path(path=w2172) -> (stripped path=w2168:path, name=w2170:string)
            n1046 = Path To String(path=w2168) -> (string=w2167:string)
            n1047 = Concatenate Strings(w2167, "\\", "X_", w2170) -> (w2166:string)
            n1048 = String To Path(string=w2166) -> (path=w2165:path)
            n1049 = Move(source path=w2172, 10:w2165) -> ()  [unwired: 3 in, 3 out]
            n1050 = local write "Data File"(w2165) -> ()
          }
          event "Cancel Button": Mouse Down {
            (unwired) 6
            n1051 = event-data() -> ()  [unwired: 1 in, 7 out]
            n1052 = call "Simulate_Keyboard.vi"("Action"=2, "Virtual Key"=162) -> ()  [unwired: 7 in, 1 out]
          }
        }
        n1053 = Reciprocal(x=w476) -> (1/x=w475:sgl)
        n1054 = Multiply(x=w475, y=10) -> (x*y=w477:sgl)
        n1055 = case shown="\"EQUALS\"" w516 {
          tunnel: w490 -> [w565 w571 w575 w577 w581 w583 w585 w587 w589 w591 w593 w595 w597 w599 w601 w603 w605 w607 w609 w611 w613 w615 w617 w619 w621 w623 w625 w627 w629 w631 w633 w635 w637 w639 w641 w643 w645 w647 w649 w651 w653 w655 w657 w659 w661 w663 w665 w667 w669 w671 w673 w675 w677 w679 w681 w683 w685 w687 w689 w691 w693 w695 w697 w699 w701 w703 w705 w707 w709 w711 w713 w715 w717 w719 w721 w723 w725 w727 w729 w731 w733 w735 w737 w739 w741 w743 w745 w747 w749 w751 w753 w755 w757 w759 w761 w763 w765 w767 w769 w771 w773 w775 w777 w779 w781]
          tunnel: [w565 w570 w574 w577 w581 w583 w585 w587 w589 w591 w593 w595 w597 w599 w601 w603 w605 w607 w609 w611 w613 w615 w617 w619 w621 w623 w625 w627 w629 w631 w633 w635 w637 w639 w641 w643 w645 w647 w649 w651 w653 w655 w657 w659 w661 w663 w665 w667 w669 w671 w673 w675 w677 w679 w681 w683 w685 w687 w689 w691 w693 w695 w697 w699 w701 w703 w705 w707 w709 w711 w713 w715 w717 w719 w721 w723 w725 w727 w729 w731 w733 w735 w737 w739 w741 w743 w745 w747 w749 w751 w753 w755 w757 w759 w761 w763 w765 w767 w769 w771 w773 w775 w777 w779 w781] -> w515
          tunnel: w491 -> [w567 w569 w573 w579 w580 w582 w584 w586 w588 w590 w592 w594 w596 w598 w600 w602 w604 w606 w608 w610 w612 w614 w616 w618 w620 w622 w624 w626 w628 w630 w632 w634 w636 w638 w640 w642 w644 w646 w648 w650 w652 w654 w656 w658 w660 w662 w664 w666 w668 w670 w672 w674 w676 w678 w680 w682 w684 w686 w688 w690 w692 w694 w696 w698 w700 w702 w704 w706 w708 w710 w712 w714 w716 w718 w720 w722 w724 w726 w728 w730 w732 w734 w736 w738 w740 w742 w744 w746 w748 w750 w752 w754 w756 w758 w760 w762 w764 w766 w768 w770 w772 w774 w776 w778 w780]
          tunnel: [w566 w569 w573 w578 w580 w582 w584 w586 w588 w590 w592 w594 w596 w598 w600 w602 w604 w606 w608 w610 w612 w614 w616 w618 w620 w622 w624 w626 w628 w630 w632 w634 w636 w638 w640 w642 w644 w646 w648 w650 w652 w654 w656 w658 w660 w662 w664 w666 w668 w670 w672 w674 w676 w678 w680 w682 w684 w686 w688 w690 w692 w694 w696 w698 w700 w702 w704 w706 w708 w710 w712 w714 w716 w718 w720 w722 w724 w726 w728 w730 w732 w734 w736 w738 w740 w742 w744 w746 w748 w750 w752 w754 w756 w758 w760 w762 w764 w766 w768 w770 w772 w774 w776 w778 w780] -> w514
          tunnel: w477 -> [w564 w568 w572 w576 _ _ _ _ _ _ _ _ _ _ _ _ _ _ _ _ _ _ _ _ _ _ _ _ _ _ _ _ _ _ _ _ _ _ _ _ _ _ _ _ _ _ _ _ _ _ _ _ _ _ _ _ _ _ _ _ _ _ _ _ _ _ _ _ _ _ _ _ _ _ _ _ _ _ _ _ _ _ _ _ _ _ _ _ _ _ _ _ _ _ _ _ _ _ _ _ _ _ _ _ _]
          frame "DOWN" {
            n1056 = Add(x=w567, y=w564) -> (x+y=w566:sgl)
          }
          frame "LEFT" {
            n1057 = Subtract(x=w571, y=w568) -> (x-y=w570:sgl)
          }
          frame "RIGHT" {
            n1058 = Add(x=w575, y=w572) -> (x+y=w574:sgl)
          }
          frame "UP" {
            n1059 = Subtract(x=w579, y=w576) -> (x-y=w578:sgl)
          }
          frame "ENTER (num pad)" {
          }
          frame "' (quote)" {
          }
          frame "END" {
          }
          frame "EQUALS" {
          }
          frame "ESCAPE" {
          }
          frame "GRAVE (`)" {
          }
          frame "HOME" {
          }
          frame "INSERT" {
          }
          frame "LBRACKET" {
          }
          frame "LCONTROL" {
          }
          frame "L ALT" {
          }
          frame "LSHIFT" {
          }
          frame "LWIN" {
          }
          frame "MINUS" {
          }
          frame "MULTIPLY" {
          }
          frame "NEXT" {
          }
          frame "NUMLOCK" {
          }
          frame "NUMPAD_0" {
          }
          frame "NUMPAD_1" {
          }
          frame "NUMPAD_2" {
          }
          frame "NUMPAD_3" {
          }
          frame "NUMPAD_4" {
          }
          frame "NUMPAD_5" {
          }
          frame "NUMPAD_6" {
          }
          frame "NUMPAD_7" {
          }
          frame "NUMPAD_8" {
          }
          frame "NUMPAD_9" {
          }
          frame "PAUSE" {
          }
          frame "PERIOD" {
          }
          frame "PRIOR (PG UP)" {
          }
          frame "RBRACKET" {
          }
          frame "RCONTROL" {
          }
          frame "RETURN" {
          }
          frame "R ALT" {
          }
          frame "RSHIFT" {
          }
          frame "RWIN" {
          }
          frame "SCROLL" {
          }
          frame "SEMICOLON" {
          }
          frame "SLASH" {
          }
          frame "SPACE" {
          }
          frame "SUBTRACT" {
          }
          frame "TAB" {
          }
          frame "DIVIDE" {
          }
          frame "DELETE" {
          }
          frame "DECIMAL" {
          }
          frame "COMMA" {
          }
          frame "CAPITAL" {
          }
          frame "BACKSLASH" {
          }
          frame "BACK" {
          }
          frame "ADD" {
          }
          frame "F15" {
          }
          frame "F14" {
          }
          frame "F13" {
          }
          frame "F12" {
          }
          frame "F11" {
          }
          frame "F10" {
          }
          frame "F9" {
          }
          frame "F8" {
          }
          frame "F7" {
          }
          frame "F6" {
          }
          frame "F5" {
          }
          frame "F4" {
          }
          frame "F3" {
          }
          frame "F2" {
          }
          frame "F1" {
          }
          frame "Z" {
          }
          frame "Y" {
          }
          frame "X" {
          }
          frame "W" {
          }
          frame "V" {
          }
          frame "U" {
          }
          frame "T" {
          }
          frame "S" {
          }
          frame "R" {
          }
          frame "Q" {
          }
          frame "P" {
          }
          frame "O" {
          }
          frame "N" {
          }
          frame "M" {
          }
          frame "L" {
          }
          frame "K" {
          }
          frame "J" {
          }
          frame "I" {
          }
          frame "H" {
          }
          frame "G" {
          }
          frame "F" {
          }
          frame "E" {
          }
          frame "D" {
          }
          frame "C" {
          }
          frame "B" {
          }
          frame "A" {
          }
          frame "9" {
          }
          frame "8" {
          }
          frame "7" {
          }
          frame "6" {
          }
          frame "5" {
          }
          frame "4" {
          }
          frame "3" {
          }
          frame "2" {
          }
          frame "1" {
          }
          frame "0" {
          }
        }
        n1060 = Bundle(w493, w492, w507, w506, 0.0) -> (w505:cluster{dbl, dbl, dbl, dbl, dbl})  [unwired: 1 in]
        n1061 = Bundle("X"=w515, "Y"=w514) -> (w509:cluster{"X":sgl, "Y":sgl})  [unwired: 1 in]
        n1062 = Divide(x=20, y=w476) -> (x/y=w479:sgl)
        n1063 = property on="Image Out" class="ImageControl"("Image Center Position"=w509) -> ()  [unwired: 2 in, 2 out]
        n1064 = call "IMAQ Convert Rectangle to ROI (Polygon)"("Rectangle"=w505) -> ("ROI Descriptor"=w503:T3)  [unwired: 7 in, 2 out]
        n1065 = Bundle("Application Font", w479, w483, w483, w483, w483, w483, TRUE, w481) -> (w485:T12)  [unwired: 1 in]
        n1066 = property on="Image Out 2" class="ImageControl"("ROI"=w503) -> ()  [unwired: 2 in, 2 out]
        n1067 = Bundle(w481, w485, w481, w481) -> (w484:T13)  [unwired: 1 in]
        n1068 = property on="Image Out" class="ImageControl"() -> ("ROI"=w458:T6)  [unwired: 2 in, 2 out]
        n1069 = Unbundle By Name(w458) -> ("Contours"=w532:T9)
        n1070 = local read "Image Out"() -> (w487:T2)
        n1071 = call "IMAQ Clear Overlay"("Image"=w487) -> ("Image Out"=w486:T2)  [unwired: 9 in, 1 out]
        n1072 = Initialize Array(0) -> (w530:i32[])  [unwired: 1 in]
        n1073 = local read "Magnification"() -> (w521:u16)
        n1074 = Array Size(array=w532) -> (size(s)=w531:i32)
        n1075 = Build Array(0.505025, 0.252522, 0.127742, 0.050345, 0.031129) -> (w522:dbl[])
        n1076 = Array Subset(array=w522, index=w521, length=1) -> (w519:dbl[])
        n1077 = property on="Image Out" class="ImageControl"() -> ("ZoomInteger"=w511:cluster{"X":i32, "Y":i32})  [unwired: 2 in, 2 out]
        n1078 = To Double Precision Float(number=w519) -> (double precision float=w518:dbl[])
        n1079 = for {
          N: w531 -> [_]
          shift-right: [w804] -> _
          shift-left: w532 -> [w804]
          shift-right: [w802] -> w517
          shift-left: w530 -> [w801]
          tunnel: w518 -> [w800]
          shift-right: [w797] -> _
          shift-left: w486 -> [w799]
          tunnel: w484 -> [w792]
          i -> [w796]
          n1080 = Index Array(array=w804, index=w796) -> (element=w813:T14)
          n1081 = Unbundle(w813) -> ("Points"=w812:i32[])  [unwired: 2 out]
          n1082 = Array To Cluster(array=w812) -> (cluster=w811:T15)
          n1083 = Unbundle(w811) -> ("Points[0]"=w791:i32, "Points[1]"=w788:i32, "Points[2]"=w803:i32, "Points[3]"=w809:i32)  [unwired: 5 out]
          n1084 = Add(x=w791, y=10) -> (x+y=w789:i32)
          n1085 = Subtract(x=w788, y=w809) -> (x-y=w808:i32)
          n1086 = Subtract(x=w791, y=w803) -> (x-y=w810:i32)
          n1087 = Square(x=w808) -> (x^2=w806:i32)
          n1088 = Square(x=w810) -> (x^2=w807:i32)
          n1089 = Add(x=w807, y=w806) -> (x+y=w805:i32)
          n1090 = Square Root(x=w805) -> (sqrt(x)=w782:dbl)
          n1091 = Multiply(x=w782, y=0.5) -> (x*y=w785:dbl)
          n1092 = Add(x=w785, y=w788) -> (x+y=w787:dbl)
          n1093 = Bundle(w789, w787) -> (w798:cluster{i32, dbl})  [unwired: 1 in]
          n1094 = Multiply(x=w782, y=w800) -> (x*y=w795:dbl[])
          n1095 = Index Array(array=w795) -> (element=w794:dbl)  [unwired: 1 in]
          n1096 = Number To Fractional String(number=w794) -> (F-format string=w793:string)  [unwired: 3 in]
          n1097 = call "IMAQ Overlay Text"("BG Color (Transparent)"=u32 0, "Text Color (black)"=u32 16448250, "Font, Size & Style"=w792, "String"=w793, "Origin"=w798, "Image"=w799) -> ("Image Out"=w797:T2)  [unwired: 4 in, 1 out]
          n1098 = Build Array (concatenate)(w801, w795) -> (w802:dbl[])
          n1099 = local write "Numeric 3"(w782) -> ()
        }
        n1100 = local write "ROI Descriptor"(w458) -> ()
        n1101 = Unbundle(w511) -> ("X"=w510:i32)  [unwired: 1 out]
        n1102 = Add Array Elements(numeric array=w517) -> (sum=w528:dbl)
        n1103 = local write "Distances"(w517) -> ()
        n1104 = local write "Total Width"(w528) -> ()
        n1105 = local write "Zoom"(w510) -> ()
        n1106 = local read "Width"() -> (w459:dbl)
        n1107 = local read "Manual"() -> (w457:bool)
        n1108 = Not(x=w457) -> (.not. x?=w455:bool)
        n1109 = local read "Total Width"() -> (w461:dbl)
        n1110 = Equal To 0?(x=w461) -> (x = 0?=w456:bool)
        n1111 = And(x=w456, y=w455) -> (x .and. y?=w454:bool)
        n1112 = case shown="True" w454 {
          tunnel: w459 -> [_ w542]
          frame False {
          }
          frame True {
            n1113 = local write "New Width"(w542) -> ()
          }
        }
        n1114 = Or(x=w456, y=w457) -> (x .or. y?=w460:bool)
        n1115 = case shown="False" w460 {
          tunnel: w461 -> [w543 _]
          frame False {
            n1116 = local write "New Width"(w543) -> ()
          }
          frame True {
          }
        }
      }
    }
  }
  n1117 = Build Array("DeviceID", "Fabricator", "Deposition", "Date", "Sample", "Row", "Column", "L (um)", "W (um)", "Material", "Treatment", "TC (mM)", "Solvent", "C (%)", "ST (C)", "Drops", "Wait (s)", "RT (F)", "RH (%)", "Ramp (s)", "RPM", "Accel (RPM/s)", "Time (s)", "Mobility", "On/Off", "Vt", "S.T.S") -> (→"Transformer \nHeaders":string[])
